vi "main.vi"() -> ()   [LabVIEW 2016]
uses:
  <vilib>/Utility/config.llb/Read Key (I32).vi
  <vilib>/Utility/config.llb/NI_LVConfig.lvlib
  <vilib>/httpClient/LabVIEWHTTPClient.lvlib
panel:
  out "QQ二维码路径":path
  out "webqq好友":string
  out "error out":errorcluster caption="错误输出"
  out "qqbat字符串":string
  out "心跳认证标志":bool
  in  "刷新时的PWM数值":dbl
  out "清扫模式记录数组":dbl[][](array[numeric])
  in  "刷新标志":bool
  out "测试布尔":bool
  out "起始秒":string
  out "起始小时":string
  out "文本已创建":bool
  out "修改定时数标志":bool
  out "错误输出 3":errorcluster caption="错误输出"
  out "布尔 2":bool
  out "清扫命令发出标志":bool
  in  "定时数":dbl=1.0
  out "图片路径":path
  in  "一直开灯":bool
  out "错误输出 2":errorcluster caption="错误输出"
  out "错误输出":errorcluster
  in  "开灯":bool
  in  "选项卡控件":T1(tab)
  in  "清扫模式选择开关":bool
  in  "清扫周期：":string="未运行"
  in  "清扫速度：":string="未运行"
  out "本机IP：":string
  out "控制器IP：":string
  in  "端口号：":i32=8848
  out "连接状态":bool
  in  "连接控制器":bool
  in  "确认定时":bool
  in  "清扫周期：":dbl(ring)=2.0 caption="清扫周期： 2" items=["2小时"=2.0, "4小时"=4.0, "6小时"=6.0, "8小时"=8.0, "10小时"=10.0, "12小时"=12.0, "14小时"=14.0]
  in  "清扫速度：":i32(slide) scale=1.0..10.0
  in  "清扫速度确认":bool
  in  "当前城市":string="杭州"
  out "天气：":string="未知"
  in  "等待：":i32=1000
  in  "断开连接":bool
  in  "确定当前城市":bool
  out "天气图标":T2
  out "滑动杆":T3 scale=0.0..100.0
  in  "清空接收区按钮":bool
  in  "待发送数据":string
  in  "发送按钮":bool
  out "数据接收显示":string="下列为接收到的数据..."
  in  "其他类清扫周期：":dbl(ring)=2.0 caption="清扫周期： 2" items=["2小时"=2.0, "4小时"=4.0, "6小时"=6.0, "8小时"=8.0, "10小时"=10.0, "12小时"=12.0, "14小时"=14.0]
  in  "其他类清扫速度：":i32(slide) scale=1.0..10.0
  in  "智能清扫模式确定按钮":bool
  in  "雨类清扫周期：":dbl(ring)=2.0 caption="清扫周期： 2" items=["2小时"=2.0, "4小时"=4.0, "6小时"=6.0, "8小时"=8.0, "10小时"=10.0, "12小时"=12.0, "14小时"=14.0]
  in  "雨类清扫速度：":i32(slide) scale=1.0..10.0
  in  "沙尘类清扫周期：":dbl(ring)=2.0 caption="清扫周期： 2" items=["2小时"=2.0, "4小时"=4.0, "6小时"=6.0, "8小时"=8.0, "10小时"=10.0, "12小时"=12.0, "14小时"=14.0]
  in  "沙尘类清扫速度：":i32(slide) scale=1.0..10.0
  in  "雪类清扫周期：":dbl(ring)=2.0 caption="清扫周期： 2" items=["2小时"=2.0, "4小时"=4.0, "6小时"=6.0, "8小时"=8.0, "10小时"=10.0, "12小时"=12.0, "14小时"=14.0]
  in  "雪类清扫速度：":i32(slide) scale=1.0..10.0
  in  "阴类清扫周期：":dbl(ring)=2.0 caption="清扫周期： 2" items=["2小时"=2.0, "4小时"=4.0, "6小时"=6.0, "8小时"=8.0, "10小时"=10.0, "12小时"=12.0, "14小时"=14.0]
  in  "阴类清扫速度：":i32(slide) scale=1.0..10.0
  in  "晴类清扫周期：":dbl(ring)=2.0 caption="清扫周期： 2" items=["2小时"=2.0, "4小时"=4.0, "6小时"=6.0, "8小时"=8.0, "10小时"=10.0, "12小时"=12.0, "14小时"=14.0]
  in  "晴类清扫速度：":i32(slide) scale=1.0..10.0
  in  "WebBrowser":refnum<k7>(container) caption="使用说明网页"
  in  "查看项目主页按钮":bool
  out "正在加载标志":T4
  in  "确认发送实时日志":bool
  out "QQ状态":bool
  out "接受者ID":string
  in  "搜索ID按钮":bool
  in  "接收者的QQ昵称或备注名":string
  in  "退出QQ号按钮":bool
  in  "打开QQ按钮":bool
  out "QQ登录二维码":picture
  out "发送返回值":string
  # "工作状态模拟"
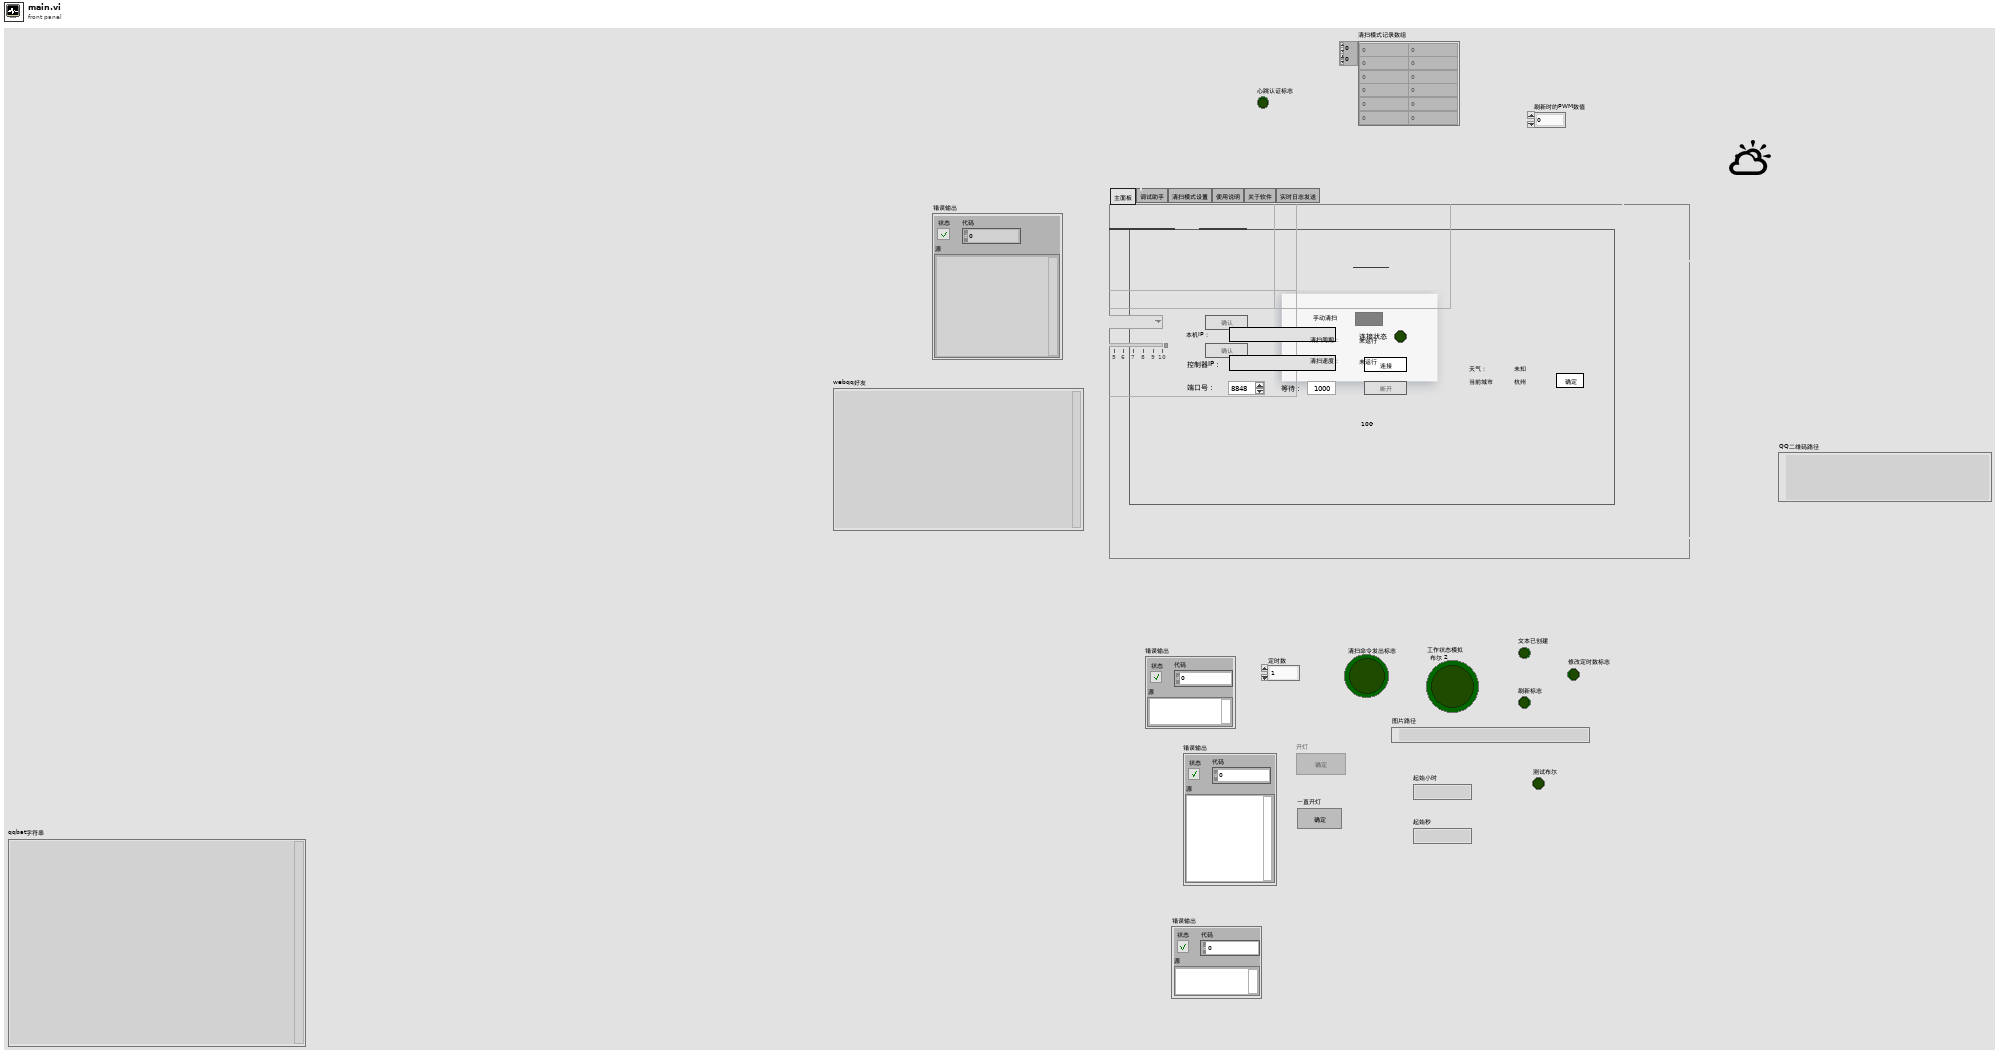
[diagram p1: front panel]
types:
  T1 = enum32{"主面板", "调试助手", "清扫模式设置", "使用说明", "关于软件", "实时日志发送"}
  T2 = typedef "透明背景.ctl" = picture
  T3 = typedef "背景控件.ctl" = dbl
  T4 = typedef "正在加载.ctl" = bool
  T5 = enum8{"Enabled", "Disabled", "Disabled and Grayed Out"}
  T6 = typedef "NI_LVConfig.lvlib/Config Data RefNum.ctl" = refnum<k1>
  T7 = typedef "LabVIEWHTTPClient.lvlib/ClientHandle.ctl" = refnum<k1>
  T8 = typedef "imagedata.ctl" = cluster{"image type":i32, "image depth":i32, "image":u8[], "mask":u8[], "colors":u32[], "Rectangle":cluster{"left":i16, "top":i16, "right":i16, "bottom":i16}}
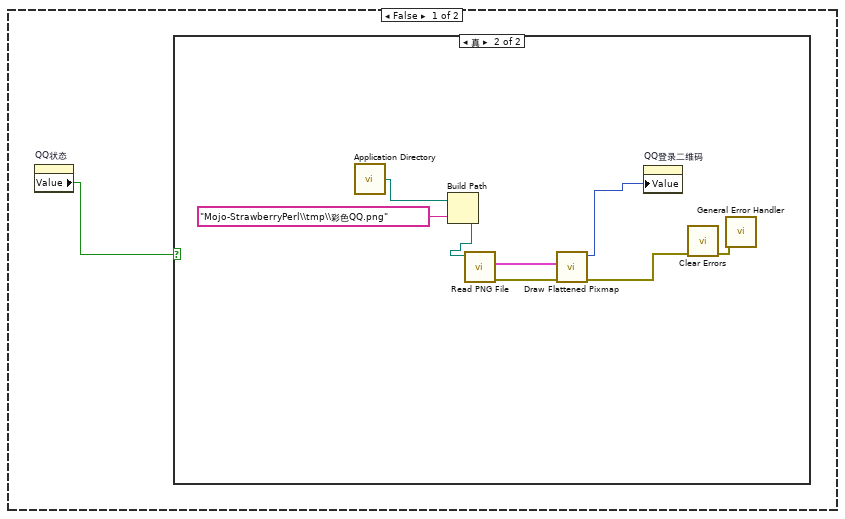
[diagram p2: hidden frame]
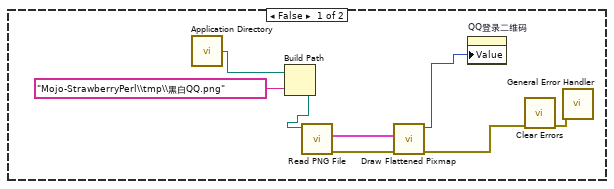
[diagram p3: hidden frame]
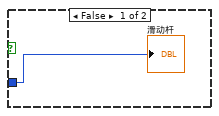
[diagram p5: hidden frame]
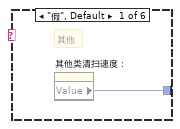
[diagram p8: hidden frame]
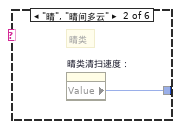
[diagram p9: hidden frame]
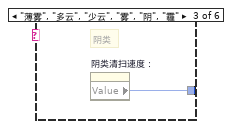
[diagram p10: hidden frame]
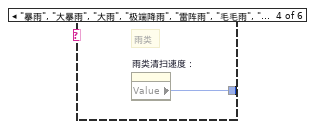
[diagram p11: hidden frame]
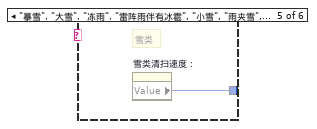
[diagram p12: hidden frame]
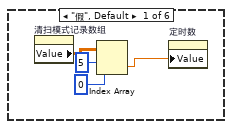
[diagram p14: hidden frame]
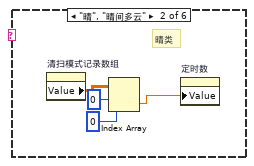
[diagram p15: hidden frame]
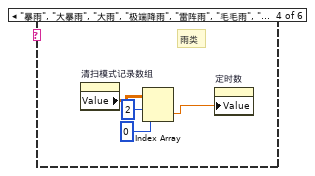
[diagram p16: hidden frame]
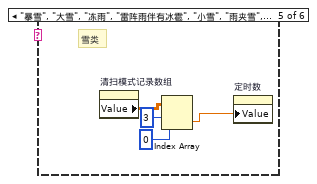
[diagram p17: hidden frame]
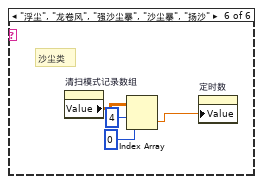
[diagram p18: hidden frame]
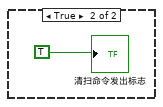
[diagram p20: hidden frame]
diagram:
  # "初始化"
  n1 = flat-sequence {
    frame #0 {
      w5 = T5."Disabled and Grayed Out" ("禁用")
      w34 = "" ("控制器IP：")
      n2 = property on="接收者的QQ昵称或备注名" class="Str"("Value"="" ("接收者的QQ昵称或备注名")) -> ()  [unwired: 2 in, 2 out]
      n3 = property on="接受者ID" class="Str"("Value"="" ("接受者ID")) -> ()  [unwired: 2 in, 2 out]
      n4 = property on="当前城市" class="Str"() -> ("Value"=w32:string)  [unwired: 2 in, 2 out]
      n5 = local write "连接状态"(FALSE ("连接状态")) -> ()
      n6 = Wait (ms)(milliseconds to wait=u32 10 ("等待时间（毫秒）")) -> ()  [unwired: 1 out]
      n7 = property on="QQ状态" class="Bool (严格)"("Value"=FALSE ("QQ状态")) -> ()  [unwired: 2 in, 2 out]
      n8 = property on="发送返回值" class="Str"("Value"="" ("发送返回值")) -> ()  [unwired: 2 in, 2 out]
      n9 = local write "本机IP："(w34) -> ()
      n10 = local write "控制器IP："(w34) -> ()
      n11 = property on="待发送数据" class="Str"("Value"="" ("待发送数据")) -> ()  [unwired: 2 in, 2 out]
      n12 = call "抓取天气查询.vi"("城市（市，县）"=w32) -> ("当前天气"=w31:string)
      n13 = property on="清扫速度：" class="Str"("Value"="未连接" ("清扫速度：")) -> ()  [unwired: 2 in, 2 out]
      n14 = property on="清扫周期：" class="Str"("Value"="未运行" ("清扫周期：")) -> ()  [unwired: 2 in, 2 out]
      n15 = call "获取时间.vi"() -> ("当前秒"=→"起始秒":string, "当前小时数"=→"起始小时":string)  [unwired: 8 in, 2 out]
      n16 = property on="天气：" class="Str"("Value"=w31) -> ()  [unwired: 2 in, 2 out]
      n17 = property on="连接控制器" class="Bool"("DisabledEnum"=T5."Enabled" ("禁用")) -> ()  [unwired: 2 in, 2 out]
      n18 = property on="正在加载标志" class="Bool (严格)"("Value"=FALSE ("获取好友标志")) -> ()  [unwired: 2 in, 2 out]
      n19 = property on="确认发送实时日志" class="Bool (严格)"("Value"=FALSE ("确认发送实时日志")) -> ()  [unwired: 2 in, 2 out]
      n20 = Concatenate Strings("和风天气图标\\" ("字符串"), "未知" ("字符串"), ".png" ("字符串")) -> (w25:string)
      n21 = property on="数据接收显示" class="Str"("Value"="下列为接收到的数据..." ("数据接收显示")) -> ()  [unwired: 2 in, 2 out]
      n22 = call <vilib>:"Application Directory.vi"() -> ("Application Directory"=w26:path)
      n23 = Initialize Array(0.0 ("元素"), 6 ("维数大小"), 2 ("维数大小")) -> (→"清扫模式记录数组":dbl[][])
      n24 = Build Path(base path=w26, name or relative path=w25) -> (appended path=w27:path)
      n25 = property on="开灯" class="Bool"("DisabledEnum"=w5) -> ()  [unwired: 2 in, 2 out]
      n26 = property on="智能清扫模式确定按钮" class="Bool"("DisabledEnum"=w5) -> ()  [unwired: 2 in, 2 out]
      n27 = property on="断开连接" class="Bool"("DisabledEnum"=w5) -> ()  [unwired: 2 in, 2 out]
      n28 = property on="发送按钮" class="Bool"("DisabledEnum"=w5) -> ()  [unwired: 2 in, 2 out]
      n29 = property on="清扫周期：" class="Ring (严格)"("DisabledEnum"=w5) -> ()  [unwired: 2 in, 2 out]
      n30 = property on="清扫速度：" class="Slide (严格)"("DisabledEnum"=w5) -> ()  [unwired: 2 in, 2 out]
      n31 = property on="确认定时" class="Bool"("DisabledEnum"=w5) -> ()  [unwired: 2 in, 2 out]
      n32 = property on="清扫速度确认" class="Bool"("DisabledEnum"=w5) -> ()  [unwired: 2 in, 2 out]
      n33 = property on="正在加载标志" class="Bool (严格)"("Visible"=FALSE ("可见")) -> ()  [unwired: 2 in, 2 out]
      n34 = property on="正在加载标志" class="Bool (严格)"("Value"=T4 FALSE ("正在加载标志")) -> ()  [unwired: 2 in, 2 out]
      n35 = property on="接收者的QQ昵称或备注名" class="Str"("DisabledEnum"=w5) -> ()  [unwired: 2 in, 2 out]
      n36 = property on="搜索ID按钮" class="Bool"("DisabledEnum"=w5) -> ()  [unwired: 2 in, 2 out]
      n37 = property on="确认发送实时日志" class="Bool (严格)"("DisabledEnum"=w5) -> ()  [unwired: 2 in, 2 out]
      n38 = property on="退出QQ号按钮" class="Bool"("DisabledEnum"=w5) -> ()  [unwired: 2 in, 2 out]
      n39 = call "显示图片.vi"("路径"=w27, "缩放因子"=1.1) -> ("二维图片"=w21:T2)  [unwired: 8 in]
      n40 = property on="天气图标" class="Pict (严格)"("Value"=w21) -> ()  [unwired: 2 in, 2 out]
    }
    frame #1 {
      n41 = call <vilib>:"Application Directory.vi"() -> ("Application Directory"=w46:path)
      n42 = Build Path(base path=w46, name or relative path="配置文件" ("名称或相对路径")) -> (appended path=w44:path)
      n43 = call <vilib>:"Open Config Data.vi"("create file if necessary (T)"=FALSE, "configuration file path"=w44) -> ("error out"=w36:errorcluster, "refnum"=w41:T6)  [unwired: 7 in, 1 out]
      n44 = call-poly <vilib>:"Read Key.vi"("section"="用户配置数据", "error in (no error)"=w36, "key"="端口号", "refnum"=w41) -> ("error out"=w37:errorcluster, "found?"=w38:bool)  [unwired: 4 in, 2 out]
      "文本已创建" <- w38
      n45 = case shown="真" w38 {
        frame False {
          n46 = call "保存配置.vi"() -> ()  [unwired: 20 in]
        }
        frame True {
        }
      }
      n47 = call <vilib>:"Clear Errors.vi"("error in (no error)"=w37) -> ("error out"=w42:errorcluster)  [unwired: 5 in, 1 out]
      n48 = call <vilib>:"General Error Handler.vi"("error in (no error)"=w42) -> ()  [unwired: 10 in, 5 out]
    }
    frame #2 {
      n49 = call "读取配置.vi"() -> ("端口号"=w51:i32, "等待"=w52:i32, "当前城市"=w53:string, "手动清扫周期"=w54:dbl, "手动清扫速度"=w55:i32, "清扫模式选择开关"=w56:bool, "晴类清扫周期"=w50:dbl, "阴类清扫周期"=w57:dbl, "雨类清扫周期"=w49:dbl, "雪类清扫周期"=w58:dbl, "沙尘类清扫周期"=w48:dbl, "其他类清扫周期"=w59:dbl, "晴类清扫速度"=w47:i32, "阴类清扫速度"=w60:i32, "雨类清扫速度"=w64:i32, "雪类清扫速度"=w63:i32, "沙尘类清扫速度"=w62:i32, "其他类清扫速度"=w61:i32)  [unwired: 2 in]
      n50 = property on="当前城市" class="Str"("Value"=w53) -> ()  [unwired: 2 in, 2 out]
      n51 = property on="等待：" class="DigNum (严格)"("Value"=w52) -> ()  [unwired: 2 in, 2 out]
      n52 = property on="端口号：" class="DigNum (严格)"("Value"=w51) -> ()  [unwired: 2 in, 2 out]
      n53 = property on="雪类清扫速度：" class="Slide (严格)"("Value"=w63) -> ()  [unwired: 2 in, 2 out]
      n54 = property on="沙尘类清扫速度：" class="Slide (严格)"("Value"=w62) -> ()  [unwired: 2 in, 2 out]
      n55 = property on="其他类清扫速度：" class="Slide (严格)"("Value"=w61) -> ()  [unwired: 2 in, 2 out]
      n56 = property on="阴类清扫速度：" class="Slide (严格)"("Value"=w60) -> ()  [unwired: 2 in, 2 out]
      n57 = property on="其他类清扫周期：" class="Ring (严格)"("Value"=w59) -> ()  [unwired: 2 in, 2 out]
      n58 = property on="雪类清扫周期：" class="Ring (严格)"("Value"=w58) -> ()  [unwired: 2 in, 2 out]
      n59 = property on="阴类清扫周期：" class="Ring (严格)"("Value"=w57) -> ()  [unwired: 2 in, 2 out]
      n60 = property on="清扫模式选择开关" class="Bool (严格)"("Value"=w56) -> ()  [unwired: 2 in, 2 out]
      n61 = property on="清扫速度：" class="Slide (严格)"("Value"=w55) -> ()  [unwired: 2 in, 2 out]
      n62 = property on="清扫周期：" class="Ring (严格)"("Value"=w54) -> ()  [unwired: 2 in, 2 out]
      n63 = property on="晴类清扫周期：" class="Ring (严格)"("Value"=w50) -> ()  [unwired: 2 in, 2 out]
      n64 = property on="雨类清扫周期：" class="Ring (严格)"("Value"=w49) -> ()  [unwired: 2 in, 2 out]
      n65 = property on="沙尘类清扫周期：" class="Ring (严格)"("Value"=w48) -> ()  [unwired: 2 in, 2 out]
      n66 = property on="晴类清扫速度：" class="Slide (严格)"("Value"=w47) -> ()  [unwired: 2 in, 2 out]
      n67 = property on="雨类清扫速度：" class="Slide (严格)"("Value"=w64) -> ()  [unwired: 2 in, 2 out]
    }
    frame #3 {
      w69 = 0 ("禁用的索引 (列)")
      w96 = 0 ("禁用的索引 (列)")
      w99 = 0 ("禁用的索引 (列)")
      w126 = 0 ("禁用的索引 (列)")
      w129 = 0 ("禁用的索引 (列)")
      w156 = 0 ("禁用的索引 (列)")
      w159 = 0 ("禁用的索引 (列)")
      w186 = 0 ("禁用的索引 (列)")
      w189 = 0 ("禁用的索引 (列)")
      w216 = 0 ("禁用的索引 (列)")
      w231 = 1 ("禁用的索引 (列)")
      # "获取本机IP地址"
      # "初始化天气图标"
      n68 = property on="天气：" class="Str"() -> ("Value"=w235:string)  [unwired: 2 in, 2 out]
      n69 = String To IP() -> (0:w66:u32)  [unwired: 1 in]
      n70 = String Length(string=w235) -> (length=w234:i32)
      n71 = IP To String(1:TRUE ("句点符号？(F)"), 2:w66) -> (0:→"本机IP：":string)
      n72 = property on="沙尘类清扫周期：" class="Ring (严格)"() -> ("Value"=w71:dbl)  [unwired: 2 in, 2 out]
      n73 = property on="沙尘类清扫周期：" class="Ring (严格)"() -> ("Value"=w94:dbl)  [unwired: 2 in, 2 out]
      n74 = property on="沙尘类清扫周期：" class="Ring (严格)"() -> ("Value"=w101:dbl)  [unwired: 2 in, 2 out]
      n75 = property on="沙尘类清扫周期：" class="Ring (严格)"() -> ("Value"=w124:dbl)  [unwired: 2 in, 2 out]
      n76 = property on="沙尘类清扫周期：" class="Ring (严格)"() -> ("Value"=w131:dbl)  [unwired: 2 in, 2 out]
      n77 = property on="沙尘类清扫周期：" class="Ring (严格)"() -> ("Value"=w154:dbl)  [unwired: 2 in, 2 out]
      n78 = property on="沙尘类清扫周期：" class="Ring (严格)"() -> ("Value"=w161:dbl)  [unwired: 2 in, 2 out]
      n79 = property on="沙尘类清扫周期：" class="Ring (严格)"() -> ("Value"=w184:dbl)  [unwired: 2 in, 2 out]
      n80 = property on="沙尘类清扫周期：" class="Ring (严格)"() -> ("Value"=w191:dbl)  [unwired: 2 in, 2 out]
      n81 = property on="沙尘类清扫周期：" class="Ring (严格)"() -> ("Value"=w214:dbl)  [unwired: 2 in, 2 out]
      n82 = Greater Than 0?(x=w234) -> (x > 0?=w233:bool)
      n83 = property on="雪类清扫周期：" class="Ring (严格)"() -> ("Value"=w73:dbl)  [unwired: 2 in, 2 out]
      n84 = property on="雪类清扫周期：" class="Ring (严格)"() -> ("Value"=w92:dbl)  [unwired: 2 in, 2 out]
      n85 = property on="雪类清扫周期：" class="Ring (严格)"() -> ("Value"=w103:dbl)  [unwired: 2 in, 2 out]
      n86 = property on="雪类清扫周期：" class="Ring (严格)"() -> ("Value"=w122:dbl)  [unwired: 2 in, 2 out]
      n87 = property on="雪类清扫周期：" class="Ring (严格)"() -> ("Value"=w133:dbl)  [unwired: 2 in, 2 out]
      n88 = property on="雪类清扫周期：" class="Ring (严格)"() -> ("Value"=w152:dbl)  [unwired: 2 in, 2 out]
      n89 = property on="雪类清扫周期：" class="Ring (严格)"() -> ("Value"=w163:dbl)  [unwired: 2 in, 2 out]
      n90 = property on="雪类清扫周期：" class="Ring (严格)"() -> ("Value"=w182:dbl)  [unwired: 2 in, 2 out]
      n91 = property on="雪类清扫周期：" class="Ring (严格)"() -> ("Value"=w193:dbl)  [unwired: 2 in, 2 out]
      n92 = property on="雪类清扫周期：" class="Ring (严格)"() -> ("Value"=w212:dbl)  [unwired: 2 in, 2 out]
      n93 = property on="雪类清扫速度：" class="Slide (严格)"() -> ("Value"=w227:i32)  [unwired: 2 in, 2 out]
      n94 = property on="晴类清扫速度：" class="Slide (严格)"() -> ("Value"=w221:i32)  [unwired: 2 in, 2 out]
      n95 = property on="阴类清扫速度：" class="Slide (严格)"() -> ("Value"=w223:i32)  [unwired: 2 in, 2 out]
      n96 = property on="雨类清扫速度：" class="Slide (严格)"() -> ("Value"=w225:i32)  [unwired: 2 in, 2 out]
      n97 = property on="沙尘类清扫速度：" class="Slide (严格)"() -> ("Value"=w229:i32)  [unwired: 2 in, 2 out]
      n98 = property on="雨类清扫周期：" class="Ring (严格)"() -> ("Value"=w75:dbl)  [unwired: 2 in, 2 out]
      n99 = property on="雨类清扫周期：" class="Ring (严格)"() -> ("Value"=w90:dbl)  [unwired: 2 in, 2 out]
      n100 = property on="雨类清扫周期：" class="Ring (严格)"() -> ("Value"=w105:dbl)  [unwired: 2 in, 2 out]
      n101 = property on="雨类清扫周期：" class="Ring (严格)"() -> ("Value"=w120:dbl)  [unwired: 2 in, 2 out]
      n102 = property on="雨类清扫周期：" class="Ring (严格)"() -> ("Value"=w135:dbl)  [unwired: 2 in, 2 out]
      n103 = property on="雨类清扫周期：" class="Ring (严格)"() -> ("Value"=w150:dbl)  [unwired: 2 in, 2 out]
      n104 = property on="雨类清扫周期：" class="Ring (严格)"() -> ("Value"=w165:dbl)  [unwired: 2 in, 2 out]
      n105 = property on="雨类清扫周期：" class="Ring (严格)"() -> ("Value"=w180:dbl)  [unwired: 2 in, 2 out]
      n106 = property on="雨类清扫周期：" class="Ring (严格)"() -> ("Value"=w195:dbl)  [unwired: 2 in, 2 out]
      n107 = property on="雨类清扫周期：" class="Ring (严格)"() -> ("Value"=w210:dbl)  [unwired: 2 in, 2 out]
      n108 = property on="其他类清扫周期：" class="Ring (严格)"() -> ("Value"=w68:dbl)  [unwired: 2 in, 2 out]
      n109 = property on="其他类清扫周期：" class="Ring (严格)"() -> ("Value"=w97:dbl)  [unwired: 2 in, 2 out]
      n110 = property on="其他类清扫周期：" class="Ring (严格)"() -> ("Value"=w98:dbl)  [unwired: 2 in, 2 out]
      n111 = property on="其他类清扫周期：" class="Ring (严格)"() -> ("Value"=w127:dbl)  [unwired: 2 in, 2 out]
      n112 = property on="其他类清扫周期：" class="Ring (严格)"() -> ("Value"=w128:dbl)  [unwired: 2 in, 2 out]
      n113 = property on="其他类清扫周期：" class="Ring (严格)"() -> ("Value"=w157:dbl)  [unwired: 2 in, 2 out]
      n114 = property on="其他类清扫周期：" class="Ring (严格)"() -> ("Value"=w158:dbl)  [unwired: 2 in, 2 out]
      n115 = property on="其他类清扫周期：" class="Ring (严格)"() -> ("Value"=w187:dbl)  [unwired: 2 in, 2 out]
      n116 = property on="其他类清扫周期：" class="Ring (严格)"() -> ("Value"=w188:dbl)  [unwired: 2 in, 2 out]
      n117 = property on="其他类清扫周期：" class="Ring (严格)"() -> ("Value"=w217:dbl)  [unwired: 2 in, 2 out]
      n118 = case shown="真" w233 {
        frame False {
        }
        frame True {
          n119 = property on="天气：" class="Str"() -> ("Value"=w236:string)  [unwired: 2 in, 2 out]
          n120 = Concatenate Strings("和风天气图标\\" ("字符串"), w236, ".png" ("字符串")) -> (w239:string)
          n121 = call <vilib>:"Application Directory.vi"() -> ("Application Directory"=w238:path)
          n122 = Build Path(base path=w238, name or relative path=w239) -> (appended path=w237:path)
          n123 = call "显示图片.vi"("路径"=w237, "缩放因子"=1.1) -> ("二维图片"=w243:T2)  [unwired: 8 in]
          n124 = property on="天气图标" class="Pict (严格)"("Value"=w243) -> ()  [unwired: 2 in, 2 out]
        }
      }
      n125 = property on="其他类清扫速度：" class="Slide (严格)"() -> ("Value"=w232:i32)  [unwired: 2 in, 2 out]
      n126 = property on="清扫模式记录数组" class="Arr (严格)"() -> ("Value"=w218:dbl[][])  [unwired: 2 in, 2 out]
      n127 = property on="阴类清扫周期：" class="Ring (严格)"() -> ("Value"=w77:dbl)  [unwired: 2 in, 2 out]
      n128 = property on="阴类清扫周期：" class="Ring (严格)"() -> ("Value"=w88:dbl)  [unwired: 2 in, 2 out]
      n129 = property on="阴类清扫周期：" class="Ring (严格)"() -> ("Value"=w107:dbl)  [unwired: 2 in, 2 out]
      n130 = property on="阴类清扫周期：" class="Ring (严格)"() -> ("Value"=w118:dbl)  [unwired: 2 in, 2 out]
      n131 = property on="阴类清扫周期：" class="Ring (严格)"() -> ("Value"=w137:dbl)  [unwired: 2 in, 2 out]
      n132 = property on="阴类清扫周期：" class="Ring (严格)"() -> ("Value"=w148:dbl)  [unwired: 2 in, 2 out]
      n133 = property on="阴类清扫周期：" class="Ring (严格)"() -> ("Value"=w167:dbl)  [unwired: 2 in, 2 out]
      n134 = property on="阴类清扫周期：" class="Ring (严格)"() -> ("Value"=w178:dbl)  [unwired: 2 in, 2 out]
      n135 = property on="阴类清扫周期：" class="Ring (严格)"() -> ("Value"=w197:dbl)  [unwired: 2 in, 2 out]
      n136 = property on="阴类清扫周期：" class="Ring (严格)"() -> ("Value"=w208:dbl)  [unwired: 2 in, 2 out]
      n137 = property on="晴类清扫周期：" class="Ring (严格)"() -> ("Value"=w81:dbl)  [unwired: 2 in, 2 out]
      n138 = property on="晴类清扫周期：" class="Ring (严格)"() -> ("Value"=w84:dbl)  [unwired: 2 in, 2 out]
      n139 = property on="晴类清扫周期：" class="Ring (严格)"() -> ("Value"=w111:dbl)  [unwired: 2 in, 2 out]
      n140 = property on="晴类清扫周期：" class="Ring (严格)"() -> ("Value"=w114:dbl)  [unwired: 2 in, 2 out]
      n141 = property on="晴类清扫周期：" class="Ring (严格)"() -> ("Value"=w141:dbl)  [unwired: 2 in, 2 out]
      n142 = property on="晴类清扫周期：" class="Ring (严格)"() -> ("Value"=w144:dbl)  [unwired: 2 in, 2 out]
      n143 = property on="晴类清扫周期：" class="Ring (严格)"() -> ("Value"=w171:dbl)  [unwired: 2 in, 2 out]
      n144 = property on="晴类清扫周期：" class="Ring (严格)"() -> ("Value"=w174:dbl)  [unwired: 2 in, 2 out]
      n145 = property on="晴类清扫周期：" class="Ring (严格)"() -> ("Value"=w201:dbl)  [unwired: 2 in, 2 out]
      n146 = property on="晴类清扫周期：" class="Ring (严格)"() -> ("Value"=w204:dbl)  [unwired: 2 in, 2 out]
      n147 = Replace Array Subset(array=w218, new element #1=w221, index (row) #1=0 ("索引 (行)"), index (col) #1=w231, new element #2=w223, index (row) #2=1 ("索引 (行)"), index (col) #2=w231, new element #3=w225, index (row) #3=2 ("索引 (行)"), index (col) #3=w231, new element #4=w227, index (row) #4=3 ("索引 (行)"), index (col) #4=w231, new element #5=w229, index (row) #5=4 ("索引 (行)"), index (col) #5=w231, new element #6=w232, index (row) #6=5 ("索引 (行)"), index (col) #6=w231) -> (w219:dbl[][])
      n148 = property on="清扫模式记录数组" class="Arr (严格)"() -> ("Value"=w82:dbl[][])  [unwired: 2 in, 2 out]
      n149 = property on="清扫模式记录数组" class="Arr (严格)"() -> ("Value"=w83:dbl[][])  [unwired: 2 in, 2 out]
      n150 = property on="清扫模式记录数组" class="Arr (严格)"() -> ("Value"=w112:dbl[][])  [unwired: 2 in, 2 out]
      n151 = property on="清扫模式记录数组" class="Arr (严格)"() -> ("Value"=w113:dbl[][])  [unwired: 2 in, 2 out]
      n152 = property on="清扫模式记录数组" class="Arr (严格)"() -> ("Value"=w142:dbl[][])  [unwired: 2 in, 2 out]
      n153 = property on="清扫模式记录数组" class="Arr (严格)"() -> ("Value"=w143:dbl[][])  [unwired: 2 in, 2 out]
      n154 = property on="清扫模式记录数组" class="Arr (严格)"() -> ("Value"=w172:dbl[][])  [unwired: 2 in, 2 out]
      n155 = property on="清扫模式记录数组" class="Arr (严格)"() -> ("Value"=w173:dbl[][])  [unwired: 2 in, 2 out]
      n156 = property on="清扫模式记录数组" class="Arr (严格)"() -> ("Value"=w202:dbl[][])  [unwired: 2 in, 2 out]
      n157 = property on="清扫模式记录数组" class="Arr (严格)"() -> ("Value"=w203:dbl[][])  [unwired: 2 in, 2 out]
      n158 = Replace Array Subset(array=w82, new element #1=w81, index (row) #1=0 ("索引 (行)"), index (col) #1=w69, new element #2=w77, index (row) #2=1 ("索引 (行)"), index (col) #2=w69, new element #3=w75, index (row) #3=2 ("索引 (行)"), index (col) #3=w69, new element #4=w73, index (row) #4=3 ("索引 (行)"), index (col) #4=w69, new element #5=w71, index (row) #5=4 ("索引 (行)"), index (col) #5=w69, new element #6=w68, index (row) #6=5 ("索引 (行)"), index (col) #6=w69) -> (w80:dbl[][])
      n159 = Replace Array Subset(array=w83, new element #1=w84, index (row) #1=0 ("索引 (行)"), index (col) #1=w96, new element #2=w88, index (row) #2=1 ("索引 (行)"), index (col) #2=w96, new element #3=w90, index (row) #3=2 ("索引 (行)"), index (col) #3=w96, new element #4=w92, index (row) #4=3 ("索引 (行)"), index (col) #4=w96, new element #5=w94, index (row) #5=4 ("索引 (行)"), index (col) #5=w96, new element #6=w97, index (row) #6=5 ("索引 (行)"), index (col) #6=w96) -> (w85:dbl[][])
      n160 = Replace Array Subset(array=w112, new element #1=w111, index (row) #1=0 ("索引 (行)"), index (col) #1=w99, new element #2=w107, index (row) #2=1 ("索引 (行)"), index (col) #2=w99, new element #3=w105, index (row) #3=2 ("索引 (行)"), index (col) #3=w99, new element #4=w103, index (row) #4=3 ("索引 (行)"), index (col) #4=w99, new element #5=w101, index (row) #5=4 ("索引 (行)"), index (col) #5=w99, new element #6=w98, index (row) #6=5 ("索引 (行)"), index (col) #6=w99) -> (w110:dbl[][])
      n161 = Replace Array Subset(array=w113, new element #1=w114, index (row) #1=0 ("索引 (行)"), index (col) #1=w126, new element #2=w118, index (row) #2=1 ("索引 (行)"), index (col) #2=w126, new element #3=w120, index (row) #3=2 ("索引 (行)"), index (col) #3=w126, new element #4=w122, index (row) #4=3 ("索引 (行)"), index (col) #4=w126, new element #5=w124, index (row) #5=4 ("索引 (行)"), index (col) #5=w126, new element #6=w127, index (row) #6=5 ("索引 (行)"), index (col) #6=w126) -> (w115:dbl[][])
      n162 = Replace Array Subset(array=w142, new element #1=w141, index (row) #1=0 ("索引 (行)"), index (col) #1=w129, new element #2=w137, index (row) #2=1 ("索引 (行)"), index (col) #2=w129, new element #3=w135, index (row) #3=2 ("索引 (行)"), index (col) #3=w129, new element #4=w133, index (row) #4=3 ("索引 (行)"), index (col) #4=w129, new element #5=w131, index (row) #5=4 ("索引 (行)"), index (col) #5=w129, new element #6=w128, index (row) #6=5 ("索引 (行)"), index (col) #6=w129) -> (w140:dbl[][])
      n163 = Replace Array Subset(array=w143, new element #1=w144, index (row) #1=0 ("索引 (行)"), index (col) #1=w156, new element #2=w148, index (row) #2=1 ("索引 (行)"), index (col) #2=w156, new element #3=w150, index (row) #3=2 ("索引 (行)"), index (col) #3=w156, new element #4=w152, index (row) #4=3 ("索引 (行)"), index (col) #4=w156, new element #5=w154, index (row) #5=4 ("索引 (行)"), index (col) #5=w156, new element #6=w157, index (row) #6=5 ("索引 (行)"), index (col) #6=w156) -> (w145:dbl[][])
      n164 = Replace Array Subset(array=w172, new element #1=w171, index (row) #1=0 ("索引 (行)"), index (col) #1=w159, new element #2=w167, index (row) #2=1 ("索引 (行)"), index (col) #2=w159, new element #3=w165, index (row) #3=2 ("索引 (行)"), index (col) #3=w159, new element #4=w163, index (row) #4=3 ("索引 (行)"), index (col) #4=w159, new element #5=w161, index (row) #5=4 ("索引 (行)"), index (col) #5=w159, new element #6=w158, index (row) #6=5 ("索引 (行)"), index (col) #6=w159) -> (w170:dbl[][])
      n165 = Replace Array Subset(array=w173, new element #1=w174, index (row) #1=0 ("索引 (行)"), index (col) #1=w186, new element #2=w178, index (row) #2=1 ("索引 (行)"), index (col) #2=w186, new element #3=w180, index (row) #3=2 ("索引 (行)"), index (col) #3=w186, new element #4=w182, index (row) #4=3 ("索引 (行)"), index (col) #4=w186, new element #5=w184, index (row) #5=4 ("索引 (行)"), index (col) #5=w186, new element #6=w187, index (row) #6=5 ("索引 (行)"), index (col) #6=w186) -> (w175:dbl[][])
      n166 = Replace Array Subset(array=w202, new element #1=w201, index (row) #1=0 ("索引 (行)"), index (col) #1=w189, new element #2=w197, index (row) #2=1 ("索引 (行)"), index (col) #2=w189, new element #3=w195, index (row) #3=2 ("索引 (行)"), index (col) #3=w189, new element #4=w193, index (row) #4=3 ("索引 (行)"), index (col) #4=w189, new element #5=w191, index (row) #5=4 ("索引 (行)"), index (col) #5=w189, new element #6=w188, index (row) #6=5 ("索引 (行)"), index (col) #6=w189) -> (w200:dbl[][])
      n167 = Replace Array Subset(array=w203, new element #1=w204, index (row) #1=0 ("索引 (行)"), index (col) #1=w216, new element #2=w208, index (row) #2=1 ("索引 (行)"), index (col) #2=w216, new element #3=w210, index (row) #3=2 ("索引 (行)"), index (col) #3=w216, new element #4=w212, index (row) #4=3 ("索引 (行)"), index (col) #4=w216, new element #5=w214, index (row) #5=4 ("索引 (行)"), index (col) #5=w216, new element #6=w217, index (row) #6=5 ("索引 (行)"), index (col) #6=w216) -> (w205:dbl[][])
      n168 = property on="清扫模式记录数组" class="Arr (严格)"("Value"=w219) -> ()  [unwired: 2 in, 2 out]
      n169 = property on="清扫模式记录数组" class="Arr (严格)"("Value"=w80) -> ()  [unwired: 2 in, 2 out]
      n170 = property on="清扫模式记录数组" class="Arr (严格)"("Value"=w85) -> ()  [unwired: 2 in, 2 out]
      n171 = property on="清扫模式记录数组" class="Arr (严格)"("Value"=w110) -> ()  [unwired: 2 in, 2 out]
      n172 = property on="清扫模式记录数组" class="Arr (严格)"("Value"=w115) -> ()  [unwired: 2 in, 2 out]
      n173 = property on="清扫模式记录数组" class="Arr (严格)"("Value"=w140) -> ()  [unwired: 2 in, 2 out]
      n174 = property on="清扫模式记录数组" class="Arr (严格)"("Value"=w145) -> ()  [unwired: 2 in, 2 out]
      n175 = property on="清扫模式记录数组" class="Arr (严格)"("Value"=w170) -> ()  [unwired: 2 in, 2 out]
      n176 = property on="清扫模式记录数组" class="Arr (严格)"("Value"=w175) -> ()  [unwired: 2 in, 2 out]
      n177 = property on="清扫模式记录数组" class="Arr (严格)"("Value"=w200) -> ()  [unwired: 2 in, 2 out]
      n178 = property on="清扫模式记录数组" class="Arr (严格)"("Value"=w205) -> ()  [unwired: 2 in, 2 out]
    }
  }
  n179 = while {
    shift-right: [w244] -> w1
    shift-left: refnum<k5> refnum ("connection ID") -> [w266]
    stop <- FALSE stop-if-true
    # "读取TCP数据"
    n180 = event shown="[2] \"打开QQ按钮\": 值改变" {
      selector: _ -> [_ _ _ _ _ _ _ _ _ _ _ _ _ _ _ _]
      dyn-events: _ -> [_ _ _ _ _ _ _ _ _ _ _ _ _ _ _ _]
      timeout: 50 -> [_ _ _ _ _ _ _ _ _ _ _ _ _ _ _ _]
      tunnel: w266 -> [w376 w379 _ _ _ _ w543 w551 w616 w621 w627 w629 w630 w639 w700 w715]
      tunnel: [w376 w377 _ _ _ _ w544 w550 w615 w618 w627 w629 w630 w638 w698 w714] -> w259
      tunnel: [_ _ _ _ _ _ _ _ w614 _ _ _ _ _ w699 w713] -> w258
      event Timeout {
        n181 = event-data() -> ()  [unwired: 1 in, 3 out]
      }
      event "连接控制器": Value Change {
        n182 = event-data() -> ()  [unwired: 1 in, 6 out]
        n183 = flat-sequence {
          tunnel: [w405] -> w380
          tunnel: [w404] -> w378
          tunnel: w379 -> [w395]
          frame #0 {
            w382 = T5."Disabled and Grayed Out" ("禁用")
            n184 = stacked-sequence {
              frame #0 {
                n185 = property on="当前城市" class="Str"() -> ("Value"=w386:string)  [unwired: 2 in, 2 out]
                n186 = call "抓取天气查询.vi"("城市（市，县）"=w386) -> ("当前天气"=w385:string)
                n187 = property on="天气：" class="Str"("Value"=w385) -> ()  [unwired: 2 in, 2 out]
              }
              frame #1 {
                n188 = call <vilib>:"Application Directory.vi"() -> ("Application Directory"=w394:path)
                n189 = property on="天气：" class="Str"() -> ("Value"=w387:string)  [unwired: 2 in, 2 out]
                n190 = Concatenate Strings("和风天气图标\\" ("字符串"), w387, ".png" ("字符串")) -> (w392:string)
                n191 = Build Path(base path=w394, name or relative path=w392) -> (appended path=w393:path)
                n192 = call "显示图片.vi"("路径"=w393, "缩放因子"=1.1) -> ("二维图片"=w388:T2)  [unwired: 8 in]
                n193 = property on="天气图标" class="Pict (严格)"("Value"=w388) -> ()  [unwired: 2 in, 2 out]
              }
            }
            n194 = property on="连接状态" class="Bool (严格)"("Value"=FALSE ("连接状态")) -> ()  [unwired: 2 in, 2 out]
            n195 = property on="清扫周期：" class="Str"("Value"="未运行" ("清扫周期：")) -> ()  [unwired: 2 in, 2 out]
            n196 = local write "控制器IP："("" ("控制器IP：")) -> ()
            n197 = property on="发送按钮" class="Bool"("DisabledEnum"=w382) -> ()  [unwired: 2 in, 2 out]
            n198 = property on="清扫速度确认" class="Bool"("DisabledEnum"=w382) -> ()  [unwired: 2 in, 2 out]
            n199 = property on="确认定时" class="Bool"("DisabledEnum"=w382) -> ()  [unwired: 2 in, 2 out]
            n200 = property on="开灯" class="Bool"("DisabledEnum"=w382) -> ()  [unwired: 2 in, 2 out]
            n201 = property on="连接控制器" class="Bool"("DisabledEnum"=w382) -> ()  [unwired: 2 in, 2 out]
          }
          frame #1 {
            n202 = call <vilib>:"TCP Listen.vi"("timeout ms (wait forever: -1)"="等待：", "port"="端口号：") -> ("error out"=w399:errorcluster, "remote address"=→"控制器IP：":string, "connection ID"=w404:refnum<k5>)  [unwired: 5 in, 2 out]
            n203 = Unbundle By Name(w399) -> ("status"=w396:bool)
            "布尔 2" <- w396
            n204 = case shown="真" w396 {
              tunnel: w395 -> [_ w408]
              frame False {
              }
              frame True {
                n205 = One Button Dialog(message="在等待时间内未连接上\n请确认端口号是否正确\n或机器是否已正确连接" ("消息"), button name ("OK")="好的我检查一下" ("T按钮名称（“确定”）")) -> (true=w409:bool)
                n206 = case shown="真" w409 {
                  tunnel: w408 -> [_ w410]
                  frame False {
                  }
                  frame True {
                    n207 = flat-sequence {
                      tunnel: w410 -> [w412]
                      frame #0 {
                        n208 = TCP Close Connection(connection ID=w412) -> (error out=→"错误输出 3":errorcluster)  [unwired: 2 in, 1 out]
                      }
                      frame #1 {
                        w413 = T5."Disabled and Grayed Out" ("禁用")
                        n209 = local write "控制器IP："("" ("控制器IP：")) -> ()
                        n210 = local write "连接状态"(FALSE ("连接状态")) -> ()
                        n211 = property on="连接控制器" class="Bool"("DisabledEnum"=T5."Enabled" ("禁用")) -> ()  [unwired: 2 in, 2 out]
                        n212 = property on="确认定时" class="Bool"("DisabledEnum"=w413) -> ()  [unwired: 2 in, 2 out]
                        n213 = property on="清扫速度确认" class="Bool"("DisabledEnum"=w413) -> ()  [unwired: 2 in, 2 out]
                        n214 = property on="开灯" class="Bool"("DisabledEnum"=w413) -> ()  [unwired: 2 in, 2 out]
                        n215 = property on="发送按钮" class="Bool"("DisabledEnum"=w413) -> ()  [unwired: 2 in, 2 out]
                        n216 = property on="断开连接" class="Bool"("DisabledEnum"=w413) -> ()  [unwired: 2 in, 2 out]
                      }
                    }
                  }
                }
              }
            }
            n217 = Not(x=w396) -> (.not. x?=w400:bool)
            n218 = Not A Number/Path/Refnum?(number/path/refnum=w404) -> (NaN/Path/Refnum?=w398:bool)
            n219 = Not(x=w398) -> (.not. x?=w397:bool)
            n220 = And(x=w397, y=w400) -> (x .and. y?=w405:bool)
          }
        }
        n221 = case shown="真" w380 {
          tunnel: w378 -> [w417 w419]
          tunnel: [w417 w418] -> w377
          frame False {
          }
          frame True {
            w421 = T5."Enabled" ("禁用")
            # "智能清扫为ON/真"
            # "恢复按钮使用权限"
            n222 = property on="清扫模式选择开关" class="Bool (严格)"() -> ("Value"=w420:bool)  [unwired: 2 in, 2 out]
            n223 = case shown="真" w420 {
              tunnel: [w429 w448] -> w418
              tunnel: w419 -> [w428 w449]
              frame False {
                w424 = T5."Enabled" ("禁用")
                # "手动清扫模式"
                n224 = property on="清扫速度：" class="Slide (严格)"() -> ("Value"=w433:i32)  [unwired: 2 in, 2 out]
                n225 = formula code="Y=X*15+105;"("X"=w433) -> ("Y"=w432:dbl)
                n226 = property on="智能清扫模式确定按钮" class="Bool"("DisabledEnum"=T5."Disabled and Grayed Out" ("禁用")) -> ()  [unwired: 2 in, 2 out]
                n227 = property on="清扫速度确认" class="Bool"("DisabledEnum"=w424) -> ()  [unwired: 2 in, 2 out]
                n228 = Number To Decimal String(number=w432) -> (decimal integer string=w430:string)  [unwired: 1 in]
                n229 = property on="确认定时" class="Bool"("DisabledEnum"=w424) -> ()  [unwired: 2 in, 2 out]
                n230 = property on="清扫周期：" class="Ring (严格)"("DisabledEnum"=w424) -> ()  [unwired: 2 in, 2 out]
                n231 = property on="清扫速度：" class="Slide (严格)"("DisabledEnum"=w424) -> ()  [unwired: 2 in, 2 out]
                n232 = Concatenate Strings("pwm" ("字符串"), w430) -> (w425:string)
                n233 = flat-sequence {
                  frame #0 {
                    n234 = property on="清扫周期：" class="Ring (严格)"() -> ("Value"=w434:dbl)  [unwired: 2 in, 2 out]
                    n235 = property on="定时数" class="DigNum (严格)"("Value"=w434) -> ()  [unwired: 2 in, 2 out]
                  }
                  frame #1 {
                    n236 = property on="定时数" class="DigNum (严格)"() -> ("Value"=w439:dbl)  [unwired: 2 in, 2 out]
                    n237 = Number To Fractional String(number=w439, precision (6)=i16 1 ("精度(6)")) -> (F-format string=w437:string)  [unwired: 2 in]
                    n238 = Concatenate Strings(w437, "小时" ("字符串")) -> (w436:string)
                    n239 = property on="清扫周期：" class="Str"("Value"=w436) -> ()  [unwired: 2 in, 2 out]
                  }
                }
                n240 = property on="清扫速度：" class="Str"("Value"=w425) -> ()  [unwired: 2 in, 2 out]
                n241 = TCP Write(connection ID=w428, data in=w425) -> (connection ID out=w429:refnum<k5>, error out=w427:errorcluster)  [unwired: 2 in, 1 out]
                n242 = call <vilib>:"Clear Errors.vi"("error in (no error)"=w427) -> ("error out"=w426:errorcluster)  [unwired: 5 in, 1 out]
                n243 = call <vilib>:"Simple Error Handler.vi"("error in (no error)"=w426) -> ()  [unwired: 4 in, 5 out]
              }
              frame True {
                w451 = T5."Disabled and Grayed Out" ("禁用")
                # "智能清扫模式"
                n244 = property on="天气：" class="Str"() -> ("Value"=w447:string)  [unwired: 2 in, 2 out]
                n245 = case shown="\"浮尘\", \"龙卷风\", \"强沙尘暴\", \"沙尘暴\", \"扬沙\"" w447 {
                  tunnel: [w452 w453 w454 w455 w456 w457] -> w440
                  frame "假", Default {
                    # "其他"
                    n246 = property on="其他类清扫速度：" class="Slide (严格)"() -> ("Value"=w452:i32)  [unwired: 2 in, 2 out]
                  }
                  frame "晴", "晴间多云" {
                    # "晴类"
                    n247 = property on="晴类清扫速度：" class="Slide (严格)"() -> ("Value"=w453:i32)  [unwired: 2 in, 2 out]
                  }
                  frame "薄雾", "多云", "少云", "雾", "阴", "霾" {
                    # "阴类"
                    n248 = property on="阴类清扫速度：" class="Slide (严格)"() -> ("Value"=w454:i32)  [unwired: 2 in, 2 out]
                  }
                  frame "暴雨", "大暴雨", "大雨", "极端降雨", "雷阵雨", "毛毛雨", "强雷阵雨", "强阵雨", "特大暴雨", "细雨", "小雨", "阵雨", "中雨" {
                    # "雨类"
                    n249 = property on="雨类清扫速度：" class="Slide (严格)"() -> ("Value"=w455:i32)  [unwired: 2 in, 2 out]
                  }
                  frame "暴雪", "大雪", "冻雨", "雷阵雨伴有冰雹", "小雪", "雨夹雪", "雨雪天气", "阵雪", "阵雨夹雪", "中雪" {
                    # "雪类"
                    n250 = property on="雪类清扫速度：" class="Slide (严格)"() -> ("Value"=w456:i32)  [unwired: 2 in, 2 out]
                  }
                  frame "浮尘", "龙卷风", "强沙尘暴", "沙尘暴", "扬沙" {
                    # "沙尘类"
                    n251 = property on="沙尘类清扫速度：" class="Slide (严格)"() -> ("Value"=w457:i32)  [unwired: 2 in, 2 out]
                  }
                }
                n252 = property on="智能清扫模式确定按钮" class="Bool"("DisabledEnum"=T5."Enabled" ("禁用")) -> ()  [unwired: 2 in, 2 out]
                n253 = property on="确认定时" class="Bool"("DisabledEnum"=w451) -> ()  [unwired: 2 in, 2 out]
                n254 = property on="清扫速度确认" class="Bool"("DisabledEnum"=w451) -> ()  [unwired: 2 in, 2 out]
                n255 = flat-sequence {
                  frame #0 {
                    # "处理清扫周期"
                    n256 = property on="天气：" class="Str"() -> ("Value"=w458:string)  [unwired: 2 in, 2 out]
                    n257 = case shown="\"薄雾\", \"多云\", \"少云\", \"雾\", \"阴\", \"霾\"" w458 {
                      frame "假", Default {
                        n258 = property on="其他类清扫周期：" class="Ring (严格)"() -> ("Value"=w459:dbl)  [unwired: 2 in, 2 out]
                        n259 = property on="定时数" class="DigNum (严格)"("Value"=w459) -> ()  [unwired: 2 in, 2 out]
                      }
                      frame "晴", "晴间多云" {
                        # "晴类"
                        n260 = property on="晴类清扫周期：" class="Ring (严格)"() -> ("Value"=w460:dbl)  [unwired: 2 in, 2 out]
                        n261 = property on="定时数" class="DigNum (严格)"("Value"=w460) -> ()  [unwired: 2 in, 2 out]
                      }
                      frame "薄雾", "多云", "少云", "雾", "阴", "霾" {
                        # "阴类"
                        n262 = property on="阴类清扫周期：" class="Ring (严格)"() -> ("Value"=w461:dbl)  [unwired: 2 in, 2 out]
                        n263 = property on="定时数" class="DigNum (严格)"("Value"=w461) -> ()  [unwired: 2 in, 2 out]
                      }
                      frame "暴雨", "大暴雨", "大雨", "极端降雨", "雷阵雨", "毛毛雨", "强雷阵雨", "强阵雨", "特大暴雨", "细雨", "小雨", "阵雨", "中雨" {
                        # "雨类"
                        n264 = property on="雨类清扫周期：" class="Ring (严格)"() -> ("Value"=w462:dbl)  [unwired: 2 in, 2 out]
                        n265 = property on="定时数" class="DigNum (严格)"("Value"=w462) -> ()  [unwired: 2 in, 2 out]
                      }
                      frame "暴雪", "大雪", "冻雨", "雷阵雨伴有冰雹", "小雪", "雨夹雪", "雨雪天气", "阵雪", "阵雨夹雪", "中雪" {
                        # "雪类"
                        n266 = property on="雪类清扫周期：" class="Ring (严格)"() -> ("Value"=w463:dbl)  [unwired: 2 in, 2 out]
                        n267 = property on="定时数" class="DigNum (严格)"("Value"=w463) -> ()  [unwired: 2 in, 2 out]
                      }
                      frame "浮尘", "龙卷风", "强沙尘暴", "沙尘暴", "扬沙" {
                        # "沙尘类"
                        n268 = property on="沙尘类清扫周期：" class="Ring (严格)"() -> ("Value"=w464:dbl)  [unwired: 2 in, 2 out]
                        n269 = property on="定时数" class="DigNum (严格)"("Value"=w464) -> ()  [unwired: 2 in, 2 out]
                      }
                    }
                  }
                  frame #1 {
                    n270 = property on="定时数" class="DigNum (严格)"() -> ("Value"=w469:dbl)  [unwired: 2 in, 2 out]
                    n271 = Number To Fractional String(number=w469, precision (6)=i16 1 ("精度(6)")) -> (F-format string=w467:string)  [unwired: 2 in]
                    n272 = Concatenate Strings(w467, "小时" ("字符串")) -> (w466:string)
                    n273 = property on="清扫周期：" class="Str"("Value"=w466) -> ()  [unwired: 2 in, 2 out]
                  }
                }
                n274 = formula code="Y=X*15+105;"("X"=w440) -> ("Y"=w446:dbl)
                n275 = Number To Decimal String(number=w446) -> (decimal integer string=w444:string)  [unwired: 1 in]
                n276 = Concatenate Strings("pwm" ("字符串"), w444) -> (w441:string)
                n277 = property on="清扫速度：" class="Str"("Value"=w441) -> ()  [unwired: 2 in, 2 out]
                n278 = TCP Write(connection ID=w449, data in=w441) -> (connection ID out=w448:refnum<k5>, error out=w443:errorcluster)  [unwired: 2 in, 1 out]
                n279 = call <vilib>:"Clear Errors.vi"("error in (no error)"=w443) -> ("error out"=w442:errorcluster)  [unwired: 5 in, 1 out]
                n280 = call <vilib>:"Simple Error Handler.vi"("error in (no error)"=w442) -> ()  [unwired: 4 in, 5 out]
              }
            }
            n281 = property on="断开连接" class="Bool"("DisabledEnum"=w421) -> ()  [unwired: 2 in, 2 out]
            n282 = property on="开灯" class="Bool"("DisabledEnum"=w421) -> ()  [unwired: 2 in, 2 out]
            n283 = property on="发送按钮" class="Bool"("DisabledEnum"=w421) -> ()  [unwired: 2 in, 2 out]
            "连接状态" <- TRUE ("控制器状态指示")
          }
        }
      }
      event "打开QQ按钮": Value Change {
        n284 = event-data() -> ()  [unwired: 1 in, 6 out]
        n285 = stacked-sequence {
          frame #0 {
            n286 = call <vilib>:"Application Directory.vi"() -> ("Application Directory"=w471:path)
            n287 = Build Path(base path=w471, name or relative path="Mojo-StrawberryPerl\\" ("名称或相对路径")) -> (appended path=w470:path)
            n288 = Build Path(base path=w470, name or relative path="start_mojo_webqq.bat" ("名称或相对路径")) -> (appended path=w476:path)
            n289 = Path To String(path=w476) -> (string=w477:string)
            n290 = call <vilib>:"System Exec.vi"("wait until completion? (T)"=FALSE, "working directory"=w470, "command line"=w477) -> ("error out"=→"error out":errorcluster, "standard output"=→"qqbat字符串":string)  [unwired: 5 in, 2 out]
          }
          frame #1 {
            n291 = property on="正在加载标志" class="Bool (严格)"("Value"=TRUE ("获取好友标志")) -> ()  [unwired: 2 in, 2 out]
            n292 = property on="正在加载标志" class="Bool (严格)"("Visible"=TRUE ("可见")) -> ()  [unwired: 2 in, 2 out]
          }
        }
      }
      event "搜索ID按钮": Value Change {
        n293 = event-data() -> ()  [unwired: 1 in, 6 out]
        n294 = flat-sequence {
          frame #0 {
            n295 = Concatenate Strings("http://127.0.0.1:5000/openqq/get_friend_info" ("字符串")) -> (w486:string)
            n296 = call <vilib>:"OpenHandle.vi"() -> ("client handle out"=w491:T7)  [unwired: 14 in, 1 out]
            n297 = Text to UTF-8(11:w486) -> (3:w488:string)  [unwired: 2 in, 1 out]
            n298 = call <vilib>:"GET.vi"("client handle"=w491, "url"=w488) -> ("client handle out"=w490:T7, "body"=w489:string, "error out"=w485:errorcluster)  [unwired: 10 in, 1 out]
            n299 = call <vilib>:"Clear Errors.vi"("error in (no error)"=w485) -> ("error out"=w484:errorcluster)  [unwired: 5 in, 1 out]
            n300 = call <vilib>:"CloseHandle.vi"("client handle"=w490) -> ()  [unwired: 14 in, 1 out]
            n301 = call <vilib>:"General Error Handler.vi"("error in (no error)"=w484) -> ()  [unwired: 10 in, 5 out]
            n302 = UTF-8 to Text(11:w489) -> (3:w482:string)  [unwired: 2 in, 1 out]
            "webqq好友" <- w482
            n303 = String Length(string=w482) -> (length=w483:i32)
            n304 = Greater Than 0?(x=w483) -> (x > 0?=w481:bool)
            n305 = case shown="真" w481 {
              frame False {
              }
              frame True {
                n306 = property on="接收者的QQ昵称或备注名" class="Str"() -> ("Value"=w494:string)  [unwired: 2 in, 2 out]
                n307 = property on="webqq好友" class="Str"() -> ("Value"=w495:string)  [unwired: 2 in, 2 out]
                n308 = Search and Replace String(replace all?=TRUE ("替换全部？(F)"), input string=w495, search string=w494) -> (number of replacements=w493:i32)  [unwired: 5 in, 3 out]
                n309 = Greater Than 0?(x=w493) -> (x > 0?=w492:bool)
                n310 = case shown="真" w492 {
                  frame False {
                  }
                  frame True {
                    n311 = property on="webqq好友" class="Str"() -> ("Value"=w500:string)  [unwired: 2 in, 2 out]
                    n312 = property on="接收者的QQ昵称或备注名" class="Str"() -> ("Value"=w499:string)  [unwired: 2 in, 2 out]
                    n313 = Match Pattern(string=w500, regular expression=w499) -> (before substring=w497:string)  [unwired: 1 in, 3 out]
                    n314 = Search and Replace String(replace all?=TRUE ("替换全部？(F)"), input string=w497, search string="\"id\"" ("搜索字符串")) -> (number of replacements=w498:i32)  [unwired: 5 in, 3 out]
                    n315 = for {
                      N: w498 -> [w506]
                      shift-right: [w503] -> _
                      shift-left: w497 -> [w504]
                      i -> [w508]
                      n316 = Decrement(x=w506) -> (x-1=w505:i32)
                      n317 = Equal?(x=w508, y=w505) -> (x = y?=w507:bool)
                      n318 = Match Pattern(string=w504, regular expression="\"id\":" ("正则表达式")) -> (after substring=w503:string)  [unwired: 1 in, 3 out]
                      n319 = case shown="真" w507 {
                        tunnel: w503 -> [_ w511]
                        frame False {
                        }
                        frame True {
                          n320 = Match Pattern(string=w511, regular expression="," ("正则表达式")) -> (before substring=→"接受者ID":string)  [unwired: 1 in, 3 out]
                        }
                      }
                    }
                  }
                }
              }
            }
          }
          frame #1 {
          }
        }
      }
      event "退出QQ号按钮": Value Change {
        n321 = event-data() -> ()  [unwired: 1 in, 6 out]
        n322 = stacked-sequence {
          frame #0 {
            n323 = property on="正在加载标志" class="Bool (严格)"("Value"=FALSE ("获取好友标志")) -> ()  [unwired: 2 in, 2 out]
            n324 = property on="QQ状态" class="Bool (严格)"("Value"=FALSE ("QQ状态")) -> ()  [unwired: 2 in, 2 out]
            n325 = property on="webqq好友" class="Str"() -> ("Value"=w523:string)  [unwired: 2 in, 2 out]
            n326 = Match Pattern(string=w523, regular expression="\"id\":" ("正则表达式")) -> (after substring=w531:string)  [unwired: 1 in, 3 out]
            n327 = call <vilib>:"Application Directory.vi"() -> ("Application Directory"=w513:path)
            n328 = call <vilib>:"Application Directory.vi"() -> ("Application Directory"=w520:path)
            n329 = Match Pattern(string=w531, regular expression="," ("正则表达式")) -> (before substring=w533:string)  [unwired: 1 in, 3 out]
            n330 = Build Path(base path=w513, name or relative path="Mojo-StrawberryPerl\\tmp\\mojo_webqq_cookie_default.dat" ("名称或相对路径")) -> (appended path=w515:path)
            n331 = Build Path(base path=w520, name or relative path="Mojo-StrawberryPerl\\tmp\\mojo_webqq_state_default.json" ("名称或相对路径")) -> (appended path=w518:path)
            n332 = call <vilib>:"Check if File or Folder Exists.vi"("path"=w515) -> ("file or folder exists?"=w516:bool, "dup path"=w517:path)  [unwired: 8 in, 1 out]
            n333 = call <vilib>:"Check if File or Folder Exists.vi"("path"=w518) -> ("file or folder exists?"=w521:bool, "dup path"=w522:path)  [unwired: 8 in, 1 out]
            n334 = Concatenate Strings("http://127.0.0.1:5000/openqq/send_friend_message?id=" ("字符串"), w533, "&content=!stop!" ("字符串")) -> (w529:string)
            n335 = case shown="真" w521 {
              tunnel: w522 -> [_ w537]
              frame False {
              }
              frame True {
                n336 = Delete(path (use dialog)=w537) -> ()  [unwired: 4 in, 3 out]
              }
            }
            n337 = case shown="真" w516 {
              tunnel: w517 -> [_ w538]
              frame False {
              }
              frame True {
                n338 = Delete(path (use dialog)=w538) -> ()  [unwired: 4 in, 3 out]
              }
            }
            n339 = call <vilib>:"OpenHandle.vi"() -> ("client handle out"=w525:T7)  [unwired: 14 in, 1 out]
            n340 = Text to UTF-8(11:w529) -> (3:w526:string)  [unwired: 2 in, 1 out]
            n341 = call <vilib>:"GET.vi"("client handle"=w525, "url"=w526) -> ("client handle out"=w524:T7, "error out"=w527:errorcluster)  [unwired: 10 in, 2 out]
            n342 = call <vilib>:"CloseHandle.vi"("client handle"=w524) -> ()  [unwired: 14 in, 1 out]
            n343 = call <vilib>:"Clear Errors.vi"("error in (no error)"=w527) -> ()  [unwired: 5 in, 2 out]
            n344 = call <vilib>:"General Error Handler.vi"() -> ()  [unwired: 11 in, 5 out]
          }
          frame #1 {
            w539 = "" ("接收者的QQ昵称或备注名")
            w540 = T5."Disabled and Grayed Out" ("禁用")
            n345 = property on="接收者的QQ昵称或备注名" class="Str"("DisabledEnum"=w540) -> ()  [unwired: 2 in, 2 out]
            n346 = property on="搜索ID按钮" class="Bool"("DisabledEnum"=w540) -> ()  [unwired: 2 in, 2 out]
            n347 = property on="确认发送实时日志" class="Bool (严格)"("DisabledEnum"=w540) -> ()  [unwired: 2 in, 2 out]
            n348 = property on="退出QQ号按钮" class="Bool"("DisabledEnum"=w540) -> ()  [unwired: 2 in, 2 out]
            n349 = property on="接收者的QQ昵称或备注名" class="Str"("Value"=w539) -> ()  [unwired: 2 in, 2 out]
            n350 = property on="接受者ID" class="Str"("Value"=w539) -> ()  [unwired: 2 in, 2 out]
          }
        }
      }
      event Panel Close? {
        n351 = event-data() -> ()  [unwired: 1 in, 4 out]
        n352 = event-data() -> ()  [unwired: 2 in, 1 out]
      }
      event "清扫速度确认": Value Change {
        n353 = event-data() -> ()  [unwired: 1 in, 6 out]
        n354 = formula code="Y=X*15+105;"("X"="清扫速度：") -> ("Y"=w542:dbl)
        n355 = Number To Decimal String(number=w542) -> (decimal integer string=w547:string)  [unwired: 1 in]
        n356 = Concatenate Strings("pwm" ("字符串"), w547) -> (w541:string)
        n357 = TCP Write(connection ID=w543, data in=w541) -> (connection ID out=w544:refnum<k5>, error out=w546:errorcluster)  [unwired: 2 in, 1 out]
        n358 = property on="清扫速度：" class="Str"("Value"=w541) -> ()  [unwired: 2 in, 2 out]
        n359 = call <vilib>:"Clear Errors.vi"("error in (no error)"=w546) -> ("error out"=w545:errorcluster)  [unwired: 5 in, 1 out]
        n360 = call <vilib>:"Simple Error Handler.vi"("error in (no error)"=w545) -> ()  [unwired: 4 in, 5 out]
      }
      event "清扫模式选择开关": Value Change {
        # "智能清扫为ON/真"
        n361 = event-data() -> ()  [unwired: 1 in, 6 out]
        n362 = case shown="真" "清扫模式选择开关" {
          tunnel: w551 -> [w554 w571]
          tunnel: [w553 w570] -> w550
          frame False {
            # "手动清扫模式"
            n363 = property on="连接状态" class="Bool (严格)"() -> ("Value"=w555:bool)  [unwired: 2 in, 2 out]
            n364 = case shown="假" w555 {
              tunnel: w554 -> [w556 w559]
              tunnel: [w556 w558] -> w553
              frame False {
                w557 = T5."Disabled and Grayed Out" ("禁用")
                n365 = property on="确认定时" class="Bool"("DisabledEnum"=w557) -> ()  [unwired: 2 in, 2 out]
                n366 = property on="清扫速度确认" class="Bool"("DisabledEnum"=w557) -> ()  [unwired: 2 in, 2 out]
                n367 = property on="清扫周期：" class="Ring (严格)"("DisabledEnum"=w557) -> ()  [unwired: 2 in, 2 out]
                n368 = property on="清扫速度：" class="Slide (严格)"("DisabledEnum"=w557) -> ()  [unwired: 2 in, 2 out]
              }
              frame True {
                w569 = T5."Enabled" ("禁用")
                n369 = property on="清扫速度：" class="Slide (严格)"() -> ("Value"=w560:i32)  [unwired: 2 in, 2 out]
                n370 = property on="确认定时" class="Bool"("DisabledEnum"=w569) -> ()  [unwired: 2 in, 2 out]
                n371 = property on="清扫速度确认" class="Bool"("DisabledEnum"=w569) -> ()  [unwired: 2 in, 2 out]
                n372 = property on="清扫周期：" class="Ring (严格)"("DisabledEnum"=w569) -> ()  [unwired: 2 in, 2 out]
                n373 = property on="清扫速度：" class="Slide (严格)"("DisabledEnum"=w569) -> ()  [unwired: 2 in, 2 out]
                n374 = formula code="Y=X*15+105;"("X"=w560) -> ("Y"=w561:dbl)
                n375 = property on="清扫周期：" class="Ring (严格)"() -> ("Value"=w568:dbl)  [unwired: 2 in, 2 out]
                n376 = property on="智能清扫模式确定按钮" class="Bool"("DisabledEnum"=T5."Disabled and Grayed Out" ("禁用")) -> ()  [unwired: 2 in, 2 out]
                n377 = Number To Decimal String(number=w561) -> (decimal integer string=w563:string)  [unwired: 1 in]
                n378 = property on="定时数" class="DigNum (严格)"("Value"=w568) -> ()  [unwired: 2 in, 2 out]
                n379 = Concatenate Strings("pwm" ("字符串"), w563) -> (w566:string)
                n380 = property on="清扫速度：" class="Str"("Value"=w566) -> ()  [unwired: 2 in, 2 out]
                n381 = TCP Write(connection ID=w559, data in=w566) -> (connection ID out=w558:refnum<k5>, error out=w564:errorcluster)  [unwired: 2 in, 1 out]
                n382 = call <vilib>:"Clear Errors.vi"("error in (no error)"=w564) -> ("error out"=w565:errorcluster)  [unwired: 5 in, 1 out]
                n383 = call <vilib>:"Simple Error Handler.vi"("error in (no error)"=w565) -> ()  [unwired: 4 in, 5 out]
              }
            }
          }
          frame True {
            # "智能清扫模式"
            n384 = property on="连接状态" class="Bool (严格)"() -> ("Value"=w572:bool)  [unwired: 2 in, 2 out]
            n385 = case shown="真" w572 {
              tunnel: w571 -> [w574 w576]
              tunnel: [w574 w575] -> w570
              frame False {
                n386 = property on="智能清扫模式确定按钮" class="Bool"("DisabledEnum"=T5."Disabled and Grayed Out" ("禁用")) -> ()  [unwired: 2 in, 2 out]
              }
              frame True {
                n387 = stacked-sequence {
                  tunnel: w576 -> [_ w588]
                  tunnel: [_ w587] -> w575
                  frame #0 {
                    n388 = flat-sequence {
                      frame #0 {
                        n389 = property on="当前城市" class="Str"() -> ("Value"=w578:string)  [unwired: 2 in, 2 out]
                        n390 = call "抓取天气查询.vi"("城市（市，县）"=w578) -> ("当前天气"=w577:string)
                        n391 = property on="天气：" class="Str"("Value"=w577) -> ()  [unwired: 2 in, 2 out]
                      }
                      frame #1 {
                        n392 = property on="天气：" class="Str"() -> ("Value"=w579:string)  [unwired: 2 in, 2 out]
                        n393 = Concatenate Strings("和风天气图标\\" ("字符串"), w579, ".png" ("字符串")) -> (w582:string)
                        n394 = call <vilib>:"Application Directory.vi"() -> ("Application Directory"=w581:path)
                        n395 = Build Path(base path=w581, name or relative path=w582) -> (appended path=w580:path)
                        n396 = call "显示图片.vi"("路径"=w580, "缩放因子"=1.1) -> ("二维图片"=w586:T2)  [unwired: 8 in]
                        n397 = property on="天气图标" class="Pict (严格)"("Value"=w586) -> ()  [unwired: 2 in, 2 out]
                      }
                    }
                  }
                  frame #1 {
                    w599 = T5."Disabled and Grayed Out" ("禁用")
                    n398 = property on="天气：" class="Str"() -> ("Value"=w596:string)  [unwired: 2 in, 2 out]
                    n399 = case shown="\"浮尘\", \"龙卷风\", \"强沙尘暴\", \"沙尘暴\", \"扬沙\"" w596 {
                      tunnel: [w600 w601 w602 w603 w604 w605] -> w589
                      frame "假", Default {
                        # "其他"
                        n400 = property on="其他类清扫速度：" class="Slide (严格)"() -> ("Value"=w600:i32)  [unwired: 2 in, 2 out]
                      }
                      frame "晴", "晴间多云" {
                        # "晴类"
                        n401 = property on="晴类清扫速度：" class="Slide (严格)"() -> ("Value"=w601:i32)  [unwired: 2 in, 2 out]
                      }
                      frame "薄雾", "多云", "少云", "雾", "阴", "霾" {
                        # "阴类"
                        n402 = property on="阴类清扫速度：" class="Slide (严格)"() -> ("Value"=w602:i32)  [unwired: 2 in, 2 out]
                      }
                      frame "暴雨", "大暴雨", "大雨", "极端降雨", "雷阵雨", "毛毛雨", "强雷阵雨", "强阵雨", "特大暴雨", "细雨", "小雨", "阵雨", "中雨" {
                        # "雨类"
                        n403 = property on="雨类清扫速度：" class="Slide (严格)"() -> ("Value"=w603:i32)  [unwired: 2 in, 2 out]
                      }
                      frame "暴雪", "大雪", "冻雨", "雷阵雨伴有冰雹", "小雪", "雨夹雪", "雨雪天气", "阵雪", "阵雨夹雪", "中雪" {
                        # "雪类"
                        n404 = property on="雪类清扫速度：" class="Slide (严格)"() -> ("Value"=w604:i32)  [unwired: 2 in, 2 out]
                      }
                      frame "浮尘", "龙卷风", "强沙尘暴", "沙尘暴", "扬沙" {
                        # "沙尘类"
                        n405 = property on="沙尘类清扫速度：" class="Slide (严格)"() -> ("Value"=w605:i32)  [unwired: 2 in, 2 out]
                      }
                    }
                    n406 = property on="天气：" class="Str"() -> ("Value"=w598:string)  [unwired: 2 in, 2 out]
                    n407 = formula code="Y=X*15+105;"("X"=w589) -> ("Y"=w595:dbl)
                    n408 = case shown="\"薄雾\", \"多云\", \"少云\", \"雾\", \"阴\", \"霾\"" w598 {
                      frame "假", Default {
                        n409 = property on="其他类清扫周期：" class="Ring (严格)"() -> ("Value"=w606:dbl)  [unwired: 2 in, 2 out]
                        n410 = property on="定时数" class="DigNum (严格)"("Value"=w606) -> ()  [unwired: 2 in, 2 out]
                      }
                      frame "晴", "晴间多云" {
                        # "晴类"
                        n411 = property on="晴类清扫周期：" class="Ring (严格)"() -> ("Value"=w607:dbl)  [unwired: 2 in, 2 out]
                        n412 = property on="定时数" class="DigNum (严格)"("Value"=w607) -> ()  [unwired: 2 in, 2 out]
                      }
                      frame "薄雾", "多云", "少云", "雾", "阴", "霾" {
                        # "阴类"
                        n413 = property on="阴类清扫周期：" class="Ring (严格)"() -> ("Value"=w608:dbl)  [unwired: 2 in, 2 out]
                        n414 = property on="定时数" class="DigNum (严格)"("Value"=w608) -> ()  [unwired: 2 in, 2 out]
                      }
                      frame "暴雨", "大暴雨", "大雨", "极端降雨", "雷阵雨", "毛毛雨", "强雷阵雨", "强阵雨", "特大暴雨", "细雨", "小雨", "阵雨", "中雨" {
                        # "雨类"
                        n415 = property on="雨类清扫周期：" class="Ring (严格)"() -> ("Value"=w609:dbl)  [unwired: 2 in, 2 out]
                        n416 = property on="定时数" class="DigNum (严格)"("Value"=w609) -> ()  [unwired: 2 in, 2 out]
                      }
                      frame "暴雪", "大雪", "冻雨", "雷阵雨伴有冰雹", "小雪", "雨夹雪", "雨雪天气", "阵雪", "阵雨夹雪", "中雪" {
                        # "雪类"
                        n417 = property on="雪类清扫周期：" class="Ring (严格)"() -> ("Value"=w610:dbl)  [unwired: 2 in, 2 out]
                        n418 = property on="定时数" class="DigNum (严格)"("Value"=w610) -> ()  [unwired: 2 in, 2 out]
                      }
                      frame "浮尘", "龙卷风", "强沙尘暴", "沙尘暴", "扬沙" {
                        # "沙尘类"
                        n419 = property on="沙尘类清扫周期：" class="Ring (严格)"() -> ("Value"=w611:dbl)  [unwired: 2 in, 2 out]
                        n420 = property on="定时数" class="DigNum (严格)"("Value"=w611) -> ()  [unwired: 2 in, 2 out]
                      }
                    }
                    n421 = property on="确认定时" class="Bool"("DisabledEnum"=w599) -> ()  [unwired: 2 in, 2 out]
                    n422 = property on="清扫速度确认" class="Bool"("DisabledEnum"=w599) -> ()  [unwired: 2 in, 2 out]
                    n423 = property on="清扫周期：" class="Ring (严格)"("DisabledEnum"=w599) -> ()  [unwired: 2 in, 2 out]
                    n424 = property on="清扫速度：" class="Slide (严格)"("DisabledEnum"=w599) -> ()  [unwired: 2 in, 2 out]
                    n425 = Number To Decimal String(number=w595) -> (decimal integer string=w593:string)  [unwired: 1 in]
                    n426 = Concatenate Strings("pwm" ("字符串"), w593) -> (w590:string)
                    n427 = property on="智能清扫模式确定按钮" class="Bool"("DisabledEnum"=T5."Enabled" ("禁用")) -> ()  [unwired: 2 in, 2 out]
                    n428 = property on="清扫速度：" class="Str"("Value"=w590) -> ()  [unwired: 2 in, 2 out]
                    n429 = TCP Write(connection ID=w588, data in=w590) -> (connection ID out=w587:refnum<k5>, error out=w592:errorcluster)  [unwired: 2 in, 1 out]
                    n430 = call <vilib>:"Clear Errors.vi"("error in (no error)"=w592) -> ("error out"=w591:errorcluster)  [unwired: 5 in, 1 out]
                    n431 = call <vilib>:"Simple Error Handler.vi"("error in (no error)"=w591) -> ()  [unwired: 4 in, 5 out]
                  }
                }
              }
            }
          }
        }
      }
      event "发送按钮": Value Change {
        n432 = event-data() -> ()  [unwired: 1 in, 6 out]
        n433 = TCP Write(connection ID=w616, data in="待发送数据", 9:500 ("超时毫秒(25000)")) -> (connection ID out=w615:refnum<k5>, error out=w614:errorcluster)  [unwired: 1 in, 1 out]
      }
      event "断开连接": Value Change {
        w617 = "未运行" ("清扫速度：")
        w619 = T5."Disabled and Grayed Out" ("禁用")
        n434 = event-data() -> ()  [unwired: 1 in, 6 out]
        n435 = TCP Close Connection(connection ID=w621) -> (connection ID out=w618:refnum<k5>, error out=→"错误输出 2":errorcluster)  [unwired: 2 in]
        n436 = local write "连接状态"(FALSE ("连接状态")) -> ()
        n437 = local write "控制器IP："("" ("控制器IP：")) -> ()
        n438 = property on="连接控制器" class="Bool"("DisabledEnum"=T5."Enabled" ("禁用")) -> ()  [unwired: 2 in, 2 out]
        n439 = property on="断开连接" class="Bool"("DisabledEnum"=w619) -> ()  [unwired: 2 in, 2 out]
        n440 = property on="清扫速度确认" class="Bool"("DisabledEnum"=w619) -> ()  [unwired: 2 in, 2 out]
        n441 = property on="确认定时" class="Bool"("DisabledEnum"=w619) -> ()  [unwired: 2 in, 2 out]
        n442 = property on="开灯" class="Bool"("DisabledEnum"=w619) -> ()  [unwired: 2 in, 2 out]
        n443 = property on="发送按钮" class="Bool"("DisabledEnum"=w619) -> ()  [unwired: 2 in, 2 out]
        n444 = property on="清扫周期：" class="Str"("Value"=w617) -> ()  [unwired: 2 in, 2 out]
        n445 = property on="清扫速度：" class="Str"("Value"=w617) -> ()  [unwired: 2 in, 2 out]
      }
      event "查看项目主页按钮": Value Change {
        n446 = event-data() -> ()  [unwired: 1 in, 6 out]
        n447 = call <vilib>:"System Exec.vi"("run minimized? (F)"=TRUE, "command line"="CMD /C start  https://github.com/skkkyoyo/Controller-of-solar-roof-cleaning-robot") -> ()  [unwired: 6 in, 4 out]
      }
      event "清空接收区按钮": Value Change {
        n448 = event-data() -> ()  [unwired: 1 in, 6 out]
        n449 = property on="数据接收显示" class="Str"("Value"="下列为接收到的数据..." ("数据接收显示")) -> ()  [unwired: 2 in, 2 out]
      }
      event "确认定时": Value Change {
        n450 = event-data() -> ()  [unwired: 1 in, 6 out]
        n451 = flat-sequence {
          frame #0 {
            n452 = property on="清扫周期：" class="Ring (严格)"() -> ("Value"=w631:dbl)  [unwired: 2 in, 2 out]
            n453 = property on="定时数" class="DigNum (严格)"("Value"=w631) -> ()  [unwired: 2 in, 2 out]
          }
          frame #1 {
            n454 = property on="定时数" class="DigNum (严格)"() -> ("Value"=w633:dbl)  [unwired: 2 in, 2 out]
            n455 = Number To Fractional String(number=w633, precision (6)=i16 1 ("精度(6)")) -> (F-format string=w635:string)  [unwired: 2 in]
            n456 = Concatenate Strings(w635, "小时" ("字符串")) -> (w636:string)
            n457 = property on="清扫周期：" class="Str"("Value"=w636) -> ()  [unwired: 2 in, 2 out]
          }
        }
      }
      event "智能清扫模式确定按钮": Value Change {
        n458 = event-data() -> ()  [unwired: 1 in, 6 out]
        n459 = flat-sequence {
          tunnel: w639 -> [w641]
          tunnel: [w640] -> w637
          tunnel: [w697] -> w638
          tunnel: w637 -> [w697]
          frame #0 {
            n460 = property on="天气：" class="Str"() -> ("Value"=w649:string)  [unwired: 2 in, 2 out]
            n461 = case shown="\"假\", 默认" w649 {
              tunnel: [w650 w651 w652 w653 w654 w655] -> w642
              frame "假", Default {
                # "其他"
                n462 = property on="其他类清扫速度：" class="Slide (严格)"() -> ("Value"=w650:i32)  [unwired: 2 in, 2 out]
              }
              frame "晴", "晴间多云" {
                # "晴类"
                n463 = property on="晴类清扫速度：" class="Slide (严格)"() -> ("Value"=w651:i32)  [unwired: 2 in, 2 out]
              }
              frame "薄雾", "多云", "少云", "雾", "阴", "霾" {
                # "阴类"
                n464 = property on="阴类清扫速度：" class="Slide (严格)"() -> ("Value"=w652:i32)  [unwired: 2 in, 2 out]
              }
              frame "暴雨", "大暴雨", "大雨", "极端降雨", "雷阵雨", "毛毛雨", "强雷阵雨", "强阵雨", "特大暴雨", "细雨", "小雨", "阵雨", "中雨" {
                # "雨类"
                n465 = property on="雨类清扫速度：" class="Slide (严格)"() -> ("Value"=w653:i32)  [unwired: 2 in, 2 out]
              }
              frame "暴雪", "大雪", "冻雨", "雷阵雨伴有冰雹", "小雪", "雨夹雪", "雨雪天气", "阵雪", "阵雨夹雪", "中雪" {
                # "雪类"
                n466 = property on="雪类清扫速度：" class="Slide (严格)"() -> ("Value"=w654:i32)  [unwired: 2 in, 2 out]
              }
              frame "浮尘", "龙卷风", "强沙尘暴", "沙尘暴", "扬沙" {
                # "沙尘类"
                n467 = property on="沙尘类清扫速度：" class="Slide (严格)"() -> ("Value"=w655:i32)  [unwired: 2 in, 2 out]
              }
            }
            n468 = flat-sequence {
              frame #0 {
                # "运行周期确认"
                n469 = property on="天气：" class="Str"() -> ("Value"=w656:string)  [unwired: 2 in, 2 out]
                n470 = case shown="\"浮尘\", \"龙卷风\", \"强沙尘暴\", \"沙尘暴\", \"扬沙\"" w656 {
                  frame "假", Default {
                    n471 = property on="其他类清扫周期：" class="Ring (严格)"() -> ("Value"=w657:dbl)  [unwired: 2 in, 2 out]
                    n472 = property on="定时数" class="DigNum (严格)"("Value"=w657) -> ()  [unwired: 2 in, 2 out]
                  }
                  frame "晴", "晴间多云" {
                    # "晴类"
                    n473 = property on="晴类清扫周期：" class="Ring (严格)"() -> ("Value"=w658:dbl)  [unwired: 2 in, 2 out]
                    n474 = property on="定时数" class="DigNum (严格)"("Value"=w658) -> ()  [unwired: 2 in, 2 out]
                  }
                  frame "薄雾", "多云", "少云", "雾", "阴", "霾" {
                    # "阴类"
                    n475 = property on="阴类清扫周期：" class="Ring (严格)"() -> ("Value"=w659:dbl)  [unwired: 2 in, 2 out]
                    n476 = property on="定时数" class="DigNum (严格)"("Value"=w659) -> ()  [unwired: 2 in, 2 out]
                  }
                  frame "暴雨", "大暴雨", "大雨", "极端降雨", "雷阵雨", "毛毛雨", "强雷阵雨", "强阵雨", "特大暴雨", "细雨", "小雨", "阵雨", "中雨" {
                    # "雨类"
                    n477 = property on="雨类清扫周期：" class="Ring (严格)"() -> ("Value"=w660:dbl)  [unwired: 2 in, 2 out]
                    n478 = property on="定时数" class="DigNum (严格)"("Value"=w660) -> ()  [unwired: 2 in, 2 out]
                  }
                  frame "暴雪", "大雪", "冻雨", "雷阵雨伴有冰雹", "小雪", "雨夹雪", "雨雪天气", "阵雪", "阵雨夹雪", "中雪" {
                    # "雪类"
                    n479 = property on="雪类清扫周期：" class="Ring (严格)"() -> ("Value"=w661:dbl)  [unwired: 2 in, 2 out]
                    n480 = property on="定时数" class="DigNum (严格)"("Value"=w661) -> ()  [unwired: 2 in, 2 out]
                  }
                  frame "浮尘", "龙卷风", "强沙尘暴", "沙尘暴", "扬沙" {
                    # "沙尘类"
                    n481 = property on="沙尘类清扫周期：" class="Ring (严格)"() -> ("Value"=w662:dbl)  [unwired: 2 in, 2 out]
                    n482 = property on="定时数" class="DigNum (严格)"("Value"=w662) -> ()  [unwired: 2 in, 2 out]
                  }
                }
              }
              frame #1 {
                n483 = property on="定时数" class="DigNum (严格)"() -> ("Value"=w666:dbl)  [unwired: 2 in, 2 out]
                n484 = Number To Decimal String(number=w666) -> (decimal integer string=w664:string)  [unwired: 1 in]
                n485 = Concatenate Strings(w664, "小时" ("字符串")) -> (w663:string)
                n486 = property on="清扫周期：" class="Str"("Value"=w663) -> ()  [unwired: 2 in, 2 out]
              }
            }
            n487 = formula code="Y=X*15+149;"("X"=w642) -> ("Y"=w648:dbl)
            n488 = Number To Decimal String(number=w648) -> (decimal integer string=w646:string)  [unwired: 1 in]
            n489 = Concatenate Strings("pwm" ("字符串"), w646) -> (w643:string)
            n490 = property on="清扫速度：" class="Str"("Value"=w643) -> ()  [unwired: 2 in, 2 out]
            n491 = TCP Write(connection ID=w641, data in=w643) -> (connection ID out=w640:refnum<k5>, error out=w645:errorcluster)  [unwired: 2 in, 1 out]
            n492 = call <vilib>:"Clear Errors.vi"("error in (no error)"=w645) -> ("error out"=w644:errorcluster)  [unwired: 5 in, 1 out]
            n493 = call <vilib>:"Simple Error Handler.vi"("error in (no error)"=w644) -> ()  [unwired: 4 in, 5 out]
          }
          frame #1 {
            w680 = 0 ("禁用的索引 (列)")
            w695 = 1 ("禁用的索引 (列)")
            n494 = property on="沙尘类清扫周期：" class="Ring (严格)"() -> ("Value"=w678:dbl)  [unwired: 2 in, 2 out]
            n495 = property on="雪类清扫周期：" class="Ring (严格)"() -> ("Value"=w676:dbl)  [unwired: 2 in, 2 out]
            n496 = property on="雨类清扫周期：" class="Ring (严格)"() -> ("Value"=w674:dbl)  [unwired: 2 in, 2 out]
            n497 = property on="其他类清扫周期：" class="Ring (严格)"() -> ("Value"=w681:dbl)  [unwired: 2 in, 2 out]
            n498 = property on="阴类清扫周期：" class="Ring (严格)"() -> ("Value"=w672:dbl)  [unwired: 2 in, 2 out]
            n499 = property on="晴类清扫周期：" class="Ring (严格)"() -> ("Value"=w668:dbl)  [unwired: 2 in, 2 out]
            n500 = property on="清扫模式记录数组" class="Arr (严格)"() -> ("Value"=w667:dbl[][])  [unwired: 2 in, 2 out]
            n501 = Replace Array Subset(array=w667, new element #1=w668, index (row) #1=0 ("索引 (行)"), index (col) #1=w680, new element #2=w672, index (row) #2=1 ("索引 (行)"), index (col) #2=w680, new element #3=w674, index (row) #3=2 ("索引 (行)"), index (col) #3=w680, new element #4=w676, index (row) #4=3 ("索引 (行)"), index (col) #4=w680, new element #5=w678, index (row) #5=4 ("索引 (行)"), index (col) #5=w680, new element #6=w681, index (row) #6=5 ("索引 (行)"), index (col) #6=w680) -> (w669:dbl[][])
            n502 = property on="雪类清扫速度：" class="Slide (严格)"() -> ("Value"=w691:i32)  [unwired: 2 in, 2 out]
            n503 = property on="晴类清扫速度：" class="Slide (严格)"() -> ("Value"=w685:i32)  [unwired: 2 in, 2 out]
            n504 = property on="阴类清扫速度：" class="Slide (严格)"() -> ("Value"=w687:i32)  [unwired: 2 in, 2 out]
            n505 = property on="雨类清扫速度：" class="Slide (严格)"() -> ("Value"=w689:i32)  [unwired: 2 in, 2 out]
            n506 = property on="沙尘类清扫速度：" class="Slide (严格)"() -> ("Value"=w693:i32)  [unwired: 2 in, 2 out]
            n507 = property on="其他类清扫速度：" class="Slide (严格)"() -> ("Value"=w696:i32)  [unwired: 2 in, 2 out]
            n508 = property on="清扫模式记录数组" class="Arr (严格)"("Value"=w669) -> ()  [unwired: 2 in, 2 out]
            n509 = property on="清扫模式记录数组" class="Arr (严格)"() -> ("Value"=w682:dbl[][])  [unwired: 2 in, 2 out]
            n510 = Replace Array Subset(array=w682, new element #1=w685, index (row) #1=0 ("索引 (行)"), index (col) #1=w695, new element #2=w687, index (row) #2=1 ("索引 (行)"), index (col) #2=w695, new element #3=w689, index (row) #3=2 ("索引 (行)"), index (col) #3=w695, new element #4=w691, index (row) #4=3 ("索引 (行)"), index (col) #4=w695, new element #5=w693, index (row) #5=4 ("索引 (行)"), index (col) #5=w695, new element #6=w696, index (row) #6=5 ("索引 (行)"), index (col) #6=w695) -> (w683:dbl[][])
            n511 = property on="清扫模式记录数组" class="Arr (严格)"("Value"=w683) -> ()  [unwired: 2 in, 2 out]
          }
        }
      }
      event "开灯": Value Change {
        n512 = event-data() -> ()  [unwired: 1 in, 6 out]
        n513 = flat-sequence {
          tunnel: [w706] -> w702
          tunnel: [w704] -> w701
          tunnel: w700 -> [w703]
          tunnel: [w709] -> w699
          tunnel: w702 -> [w710]
          tunnel: w701 -> [w712]
          tunnel: [w711] -> w698
          frame #0 {
            n514 = TCP Write(connection ID=w703, data in="ledon" ("数据输入")) -> (connection ID out=w704:refnum<k5>, error out=w706:errorcluster)  [unwired: 2 in, 1 out]
            n515 = Wait (ms)(milliseconds to wait=u32 1000 ("等待时间（毫秒）")) -> ()  [unwired: 1 out]
          }
          frame #1 {
            n516 = TCP Write(connection ID=w712, data in="ledoff" ("数据输入"), error in (no error)=w710) -> (connection ID out=w711:refnum<k5>, error out=w709:errorcluster)  [unwired: 1 in, 1 out]
          }
        }
      }
      event "一直开灯": Value Change {
        n517 = event-data() -> ()  [unwired: 1 in, 6 out]
        n518 = TCP Write(connection ID=w715, data in="ledon" ("数据输入")) -> (connection ID out=w714:refnum<k5>, error out=w713:errorcluster)  [unwired: 2 in, 1 out]
      }
    }
    n519 = property on="webqq好友" class="Str" props=["Value"]() -> ()  [unwired: 2 in, 3 out]
    n520 = property on="接收者的QQ昵称或备注名" class="Str" props=["Value"]() -> ()  [unwired: 2 in, 3 out]
    n521 = property on="清扫命令发出标志" class="Bool (严格)"() -> ("Value"=w256:bool)  [unwired: 2 in, 2 out]
    n522 = case shown="真" w256 {
      tunnel: w259 -> [w333 w339]
      tunnel: [w333 w338] -> w254
      tunnel: w258 -> [w334 w337]
      tunnel: [w334 w336] -> w257
      frame False {
      }
      frame True {
        n523 = flat-sequence {
          tunnel: w339 -> [w344]
          tunnel: w337 -> [w342]
          tunnel: [w341] -> w336
          tunnel: [w343] -> w335
          tunnel: [w348] -> w338
          tunnel: w335 -> [w348]
          frame #0 {
            n524 = TCP Write(connection ID=w344, data in="clean" ("数据输入"), error in (no error)=w342, 9:500 ("超时毫秒(25000)")) -> (connection ID out=w343:refnum<k5>, error out=w341:errorcluster)  [unwired: 1 out]
            n525 = Wait (ms)(milliseconds to wait=u32 100 ("等待时间（毫秒）")) -> ()  [unwired: 1 out]
          }
          frame #1 {
            n526 = property on="清扫命令发出标志" class="Bool (严格)"("Value"=FALSE ("清扫命令发出")) -> ()  [unwired: 2 in, 2 out]
          }
        }
      }
    }
    n527 = case shown="假" "刷新标志" {
      tunnel: w254 -> [w285 w303]
      tunnel: [w285 w301] -> w253
      frame False {
        n528 = disable-structure shown="禁用" {
          frame Disabled {
            n529 = call "获取时间.vi"() -> ("当前秒"=w292:string)  [unwired: 8 in, 3 out]
            n530 = Decimal String To Number(string=w292) -> (number=w291:i32)  [unwired: 2 in, 1 out]
            n531 = Quotient & Remainder(x=w291, y=5) -> (x-y*floor(x/y)=w289:i32)  [unwired: 1 out]
            n532 = Equal?(x=w289, y=0 ("x-y*floor(x/y)")) -> (x = y?=w287:bool)
            n533 = case shown="真" w287 {
              tunnel: [w293 w299] -> w286
              tunnel: [w293 w298] -> _
              frame False {
              }
              frame True {
                # "心跳认证"
                n534 = TCP Write(connection ID=w299, data in="heartbeat " ("数据输入")) -> (connection ID out=w298:refnum<k5>, error out=w294:errorcluster)  [unwired: 2 in, 1 out]
                n535 = call <vilib>:"Clear Errors.vi"("error in (no error)"=w294) -> ("error out"=w295:errorcluster)  [unwired: 5 in, 1 out]
                n536 = call <vilib>:"Simple Error Handler.vi"("error in (no error)"=w295) -> ()  [unwired: 4 in, 5 out]
                "心跳认证标志" <- TRUE ("心跳认证标志")
              }
            }
          }
          frame Enabled {
          }
        }
      }
      frame True {
        n537 = property on="天气：" class="Str"() -> ("Value"=w305:string)  [unwired: 2 in, 2 out]
        n538 = case shown="\"浮尘\", \"龙卷风\", \"强沙尘暴\", \"沙尘暴\", \"扬沙\"" w305 {
          frame "假", Default {
            # "其他"
            n539 = property on="清扫模式记录数组" class="Arr (严格)"() -> ("Value"=w312:dbl[][])  [unwired: 2 in, 2 out]
            n540 = Index Array(array=w312, index (row)=5 ("索引 (行)"), index (col)=1 ("禁用的索引 (列)")) -> (element=w309:dbl)
            n541 = property on="刷新时的PWM数值" class="DigNum (严格)"("Value"=w309) -> ()  [unwired: 2 in, 2 out]
          }
          frame "晴", "晴间多云" {
            # "晴类"
            n542 = property on="清扫模式记录数组" class="Arr (严格)"() -> ("Value"=w314:dbl[][])  [unwired: 2 in, 2 out]
            n543 = Index Array(array=w314, index (row)=0 ("索引 (行)"), index (col)=1 ("禁用的索引 (列)")) -> (element=w313:dbl)
            n544 = property on="刷新时的PWM数值" class="DigNum (严格)"("Value"=w313) -> ()  [unwired: 2 in, 2 out]
          }
          frame "薄雾", "多云", "少云", "雾", "阴", "霾" {
            # "阴类"
            n545 = property on="清扫模式记录数组" class="Arr (严格)"() -> ("Value"=w320:dbl[][])  [unwired: 2 in, 2 out]
            n546 = Index Array(array=w320, index (row)=1 ("索引 (行)"), index (col)=1 ("禁用的索引 (列)")) -> (element=w317:dbl)
            n547 = property on="刷新时的PWM数值" class="DigNum (严格)"("Value"=w317) -> ()  [unwired: 2 in, 2 out]
          }
          frame "暴雨", "大暴雨", "大雨", "极端降雨", "雷阵雨", "毛毛雨", "强雷阵雨", "强阵雨", "特大暴雨", "细雨", "小雨", "阵雨", "中雨" {
            # "雨类"
            n548 = property on="清扫模式记录数组" class="Arr (严格)"() -> ("Value"=w324:dbl[][])  [unwired: 2 in, 2 out]
            n549 = Index Array(array=w324, index (row)=2 ("索引 (行)"), index (col)=1 ("禁用的索引 (列)")) -> (element=w321:dbl)
            n550 = property on="刷新时的PWM数值" class="DigNum (严格)"("Value"=w321) -> ()  [unwired: 2 in, 2 out]
          }
          frame "暴雪", "大雪", "冻雨", "雷阵雨伴有冰雹", "小雪", "雨夹雪", "雨雪天气", "阵雪", "阵雨夹雪", "中雪" {
            # "雪类"
            n551 = property on="清扫模式记录数组" class="Arr (严格)"() -> ("Value"=w328:dbl[][])  [unwired: 2 in, 2 out]
            n552 = Index Array(array=w328, index (row)=3 ("索引 (行)"), index (col)=1 ("禁用的索引 (列)")) -> (element=w325:dbl)
            n553 = property on="刷新时的PWM数值" class="DigNum (严格)"("Value"=w325) -> ()  [unwired: 2 in, 2 out]
          }
          frame "浮尘", "龙卷风", "强沙尘暴", "沙尘暴", "扬沙" {
            # "沙尘类"
            n554 = property on="清扫模式记录数组" class="Arr (严格)"() -> ("Value"=w332:dbl[][])  [unwired: 2 in, 2 out]
            n555 = Index Array(array=w332, index (row)=4 ("索引 (行)"), index (col)=1 ("禁用的索引 (列)")) -> (element=w330:dbl)
            n556 = property on="刷新时的PWM数值" class="DigNum (严格)"("Value"=w330) -> ()  [unwired: 2 in, 2 out]
          }
        }
        n557 = property on="刷新标志" class="Bool (严格)"("Value"=FALSE ("刷新标志")) -> ()  [unwired: 2 in, 2 out]
        n558 = formula code="Y=X*15+105;"("X"="刷新时的PWM数值") -> ("Y"=w306:dbl)
        n559 = Number To Decimal String(number=w306) -> (decimal integer string=w308:string)  [unwired: 1 in]
        n560 = Concatenate Strings("pwm" ("字符串"), w308) -> (w304:string)
        n561 = property on="清扫速度：" class="Str"("Value"=w304) -> ()  [unwired: 2 in, 2 out]
        n562 = TCP Write(connection ID=w303, data in=w304) -> (connection ID out=w301:refnum<k5>)  [unwired: 2 in, 2 out]
      }
    }
    n563 = TCP Read(connection ID=w253, bytes to read=512, error in (no error)=w257, 9:50) -> (connection ID out=w245:refnum<k5>, data out=w263:string, error out=w252:errorcluster)  [unwired: 1 in]
    "错误输出" <- w252
    n564 = String Length(string=w263) -> (length=w261:i32)
    n565 = Greater Than 0?(x=w261) -> (x > 0?=w260:bool)
    n566 = case shown="真" w260 {
      tunnel: w263 -> [_ w351]
      frame False {
      }
      frame True {
        n567 = property on="数据接收显示" class="Str"() -> ("Value"=w358:string)  [unwired: 2 in, 2 out]
        n568 = Concatenate Strings(w358, "\r", w351) -> (w356:string)
        "数据接收显示" <- w356
        n569 = property on="待发送数据" class="Str"("Value"="" ("待发送数据")) -> ()  [unwired: 2 in, 2 out]
        n570 = String Length(string=w356) -> (length=w355:i32)
        n571 = property on="QQ状态" class="Bool (严格)"() -> ("Value"=w353:bool)  [unwired: 2 in, 2 out]
        n572 = String Length(string=w351) -> (length=w350:i32)
        n573 = property on="数据接收显示" class="Str"("Text.Scroll Position"=w355) -> ()  [unwired: 2 in, 2 out]
        n574 = Greater Than 0?(x=w350) -> (x > 0?=w349:bool)
        n575 = Compound Arithmetic op=AND ("复合运算")(w353, "确认发送实时日志", w349) -> (w354:bool)
        n576 = case shown="真" w354 {
          tunnel: w351 -> [_ w361]
          frame False {
          }
          frame True {
            # "QQ实时日志发送"
            n577 = property on="接受者ID" class="Str"() -> ("Value"=w365:string)  [unwired: 2 in, 2 out]
            n578 = call "获取时间.vi"() -> ("当前时间"=w362:string, "当前日期"=w364:string)  [unwired: 8 in, 2 out]
            n579 = Concatenate Strings("http://127.0.0.1:5000/openqq/send_friend_message?id=" ("字符串"), w365, "&content=" ("字符串"), w364, "  " ("字符串"), w362, "  " ("字符串"), w361) -> (w368:string)
            n580 = call <vilib>:"OpenHandle.vi"() -> ("client handle out"=w373:T7)  [unwired: 14 in, 1 out]
            n581 = Text to UTF-8(11:w368) -> (3:w370:string)  [unwired: 2 in, 1 out]
            n582 = call <vilib>:"GET.vi"("client handle"=w373, "url"=w370) -> ("client handle out"=w372:T7, "body"=w371:string, "error out"=w367:errorcluster)  [unwired: 10 in, 1 out]
            n583 = call <vilib>:"Clear Errors.vi"("error in (no error)"=w367) -> ("error out"=w366:errorcluster)  [unwired: 5 in, 1 out]
            n584 = call <vilib>:"CloseHandle.vi"("client handle"=w372) -> ()  [unwired: 14 in, 1 out]
            n585 = call <vilib>:"General Error Handler.vi"("error in (no error)"=w366) -> ()  [unwired: 10 in, 5 out]
            n586 = UTF-8 to Text(11:w371) -> (3:→"发送返回值":string)  [unwired: 2 in, 1 out]
          }
        }
      }
    }
    n587 = Unbundle(w252) -> ("code"=w249:i32)  [unwired: 2 out]
    n588 = Wait (ms)(milliseconds to wait=u32 50 ("等待时间（毫秒）")) -> ()  [unwired: 1 out]
    n589 = Equal?(x=66, y=w249) -> (x = y?=w248:bool)
    n590 = Equal?(x=w249, y=63) -> (x = y?=w247:bool)
    n591 = Or(x=w248, y=w247) -> (x .or. y?=w246:bool)
    n592 = case shown="真" w246 {
      tunnel: w245 -> [w269 w271]
      tunnel: [w269 w270] -> w244
      frame False {
      }
      frame True {
        n593 = One Button Dialog(message="链接似乎被中断" ("消息"), button name ("OK")="我已了解" ("按钮名称（“确定”）")) -> (true=w272:bool)
        n594 = case shown="真" w272 {
          tunnel: w271 -> [w275 w280]
          tunnel: [w275 w279] -> w270
          frame False {
          }
          frame True {
            w276 = "未运行" ("清扫速度：")
            w284 = T5."Disabled and Grayed Out" ("禁用")
            n595 = TCP Close Connection(connection ID=w280) -> (connection ID out=w279:refnum<k5>, error out=w277:errorcluster)  [unwired: 2 in]
            n596 = local write "控制器IP："("" ("控制器IP：")) -> ()
            n597 = local write "连接状态"(FALSE ("连接状态")) -> ()
            n598 = property on="清扫周期：" class="Str"("Value"=w276) -> ()  [unwired: 2 in, 2 out]
            n599 = property on="连接控制器" class="Bool"("DisabledEnum"=T5."Enabled" ("禁用")) -> ()  [unwired: 2 in, 2 out]
            n600 = call <vilib>:"Clear Errors.vi"("error in (no error)"=w277) -> ("error out"=w278:errorcluster)  [unwired: 5 in, 1 out]
            n601 = property on="清扫速度：" class="Str"("Value"=w276) -> ()  [unwired: 2 in, 2 out]
            n602 = call <vilib>:"Simple Error Handler.vi"("error in (no error)"=w278) -> ()  [unwired: 4 in, 5 out]
            n603 = property on="断开连接" class="Bool"("DisabledEnum"=w284) -> ()  [unwired: 2 in, 2 out]
            n604 = property on="清扫速度确认" class="Bool"("DisabledEnum"=w284) -> ()  [unwired: 2 in, 2 out]
            n605 = property on="确认定时" class="Bool"("DisabledEnum"=w284) -> ()  [unwired: 2 in, 2 out]
            n606 = property on="开灯" class="Bool"("DisabledEnum"=w284) -> ()  [unwired: 2 in, 2 out]
            n607 = property on="发送按钮" class="Bool"("DisabledEnum"=w284) -> ()  [unwired: 2 in, 2 out]
          }
        }
      }
    }
  }
  n608 = while {
    stop <- FALSE stop-if-true
    n609 = property on="正在加载标志" class="Bool (严格)"() -> ("Value"=w717:bool)  [unwired: 2 in, 2 out]
    n610 = case shown="真" w717 {
      frame False {
        n611 = property on="QQ状态" class="Bool (严格)"() -> ("Value"=w719:bool)  [unwired: 2 in, 2 out]
        n612 = case shown="真" w719 {
          frame False {
            n613 = call <vilib>:"Application Directory.vi"() -> ("Application Directory"=w724:path)
            n614 = Build Path(base path=w724, name or relative path="Mojo-StrawberryPerl\\tmp\\黑白QQ.png" ("名称或相对路径")) -> (appended path=w723:path)
            n615 = call <vilib>:"Read PNG File.vi"("path to PNG file"=w723) -> ("error out"=w721:errorcluster, "image data"=w726:T8)  [unwired: 8 in, 1 out]
            n616 = call <vilib>:"Draw Flattened Pixmap.vi"("image data"=w726) -> ("new picture"=w720:picture)  [unwired: 8 in]
            n617 = property on="QQ登录二维码" class="Pict"("Value"=w720) -> ()  [unwired: 2 in, 2 out]
            n618 = call <vilib>:"Clear Errors.vi"("error in (no error)"=w721) -> ("error out"=w722:errorcluster)  [unwired: 5 in, 1 out]
            n619 = call <vilib>:"General Error Handler.vi"("error in (no error)"=w722) -> ()  [unwired: 10 in, 5 out]
          }
          frame True {
            n620 = call <vilib>:"Application Directory.vi"() -> ("Application Directory"=w731:path)
            n621 = Build Path(base path=w731, name or relative path="Mojo-StrawberryPerl\\tmp\\彩色QQ.png" ("名称或相对路径")) -> (appended path=w730:path)
            n622 = call <vilib>:"Read PNG File.vi"("path to PNG file"=w730) -> ("error out"=w728:errorcluster, "image data"=w733:T8)  [unwired: 8 in, 1 out]
            n623 = call <vilib>:"Draw Flattened Pixmap.vi"("image data"=w733) -> ("new picture"=w727:picture)  [unwired: 8 in]
            n624 = property on="QQ登录二维码" class="Pict"("Value"=w727) -> ()  [unwired: 2 in, 2 out]
            n625 = call <vilib>:"Clear Errors.vi"("error in (no error)"=w728) -> ("error out"=w729:errorcluster)  [unwired: 5 in, 1 out]
            n626 = call <vilib>:"General Error Handler.vi"("error in (no error)"=w729) -> ()  [unwired: 10 in, 5 out]
          }
        }
      }
      frame True {
        n627 = call <vilib>:"Application Directory.vi"() -> ("Application Directory"=w737:path)
        n628 = Concatenate Strings("http://127.0.0.1:5000/openqq/get_friend_info" ("字符串")) -> (w749:string)
        n629 = Build Path(base path=w737, name or relative path="Mojo-StrawberryPerl\\tmp\\webqq.png" ("名称或相对路径")) -> (appended path=w736:path)
        "QQ二维码路径" <- w736
        n630 = call <vilib>:"Read PNG File.vi"("path to PNG file"=w736) -> ("error out"=w734:errorcluster, "image data"=w740:T8)  [unwired: 8 in, 1 out]
        n631 = call <vilib>:"OpenHandle.vi"() -> ("client handle out"=w744:T7)  [unwired: 14 in, 1 out]
        n632 = Text to UTF-8(11:w749) -> (3:w747:string)  [unwired: 2 in, 1 out]
        n633 = call <vilib>:"GET.vi"("client handle"=w744, "url"=w747) -> ("client handle out"=w745:T7, "body"=w746:string, "error out"=w750:errorcluster)  [unwired: 10 in, 1 out]
        n634 = call <vilib>:"Clear Errors.vi"("error in (no error)"=w750) -> ("error out"=w751:errorcluster)  [unwired: 5 in, 1 out]
        n635 = call <vilib>:"CloseHandle.vi"("client handle"=w745) -> ()  [unwired: 14 in, 1 out]
        n636 = call <vilib>:"Draw Flattened Pixmap.vi"("image data"=w740) -> ("new picture"=→"QQ登录二维码":picture)  [unwired: 8 in]
        n637 = call <vilib>:"General Error Handler.vi"("error in (no error)"=w751) -> ()  [unwired: 10 in, 5 out]
        n638 = UTF-8 to Text(11:w746) -> (3:w742:string)  [unwired: 2 in, 1 out]
        n639 = String Length(string=w742) -> (length=w743:i32)
        n640 = property on="webqq好友" class="Str"("Value"=w742) -> ()  [unwired: 2 in, 2 out]
        n641 = call <vilib>:"Clear Errors.vi"("error in (no error)"=w734) -> ("error out"=w735:errorcluster)  [unwired: 5 in, 1 out]
        n642 = Greater Than 0?(x=w743) -> (x > 0?=w741:bool)
        n643 = call <vilib>:"General Error Handler.vi"("error in (no error)"=w735) -> ()  [unwired: 10 in, 5 out]
        n644 = case shown="真" w741 {
          frame False {
          }
          frame True {
            w753 = T5."Enabled" ("禁用")
            w752 = FALSE ("获取好友标志")
            n645 = property on="接收者的QQ昵称或备注名" class="Str"("DisabledEnum"=w753) -> ()  [unwired: 2 in, 2 out]
            n646 = property on="搜索ID按钮" class="Bool"("DisabledEnum"=w753) -> ()  [unwired: 2 in, 2 out]
            n647 = property on="确认发送实时日志" class="Bool (严格)"("DisabledEnum"=w753) -> ()  [unwired: 2 in, 2 out]
            n648 = property on="退出QQ号按钮" class="Bool"("DisabledEnum"=w753) -> ()  [unwired: 2 in, 2 out]
            n649 = property on="正在加载标志" class="Bool (严格)"("Visible"=w752) -> ()  [unwired: 2 in, 2 out]
            "QQ状态" <- TRUE ("QQ状态")
            "正在加载标志" <- w752
          }
        }
      }
    }
  }
  n650 = while {
    stop <- FALSE stop-if-true
    # "选项卡切换"
    n651 = Current VI's Menubar() -> (w757:refnum<k9>)
    n652 = Get Menu Selection(0:w757) -> (6:w756:string)  [unwired: 3 in, 4 out]
    n653 = Wait (ms)(milliseconds to wait=u32 50 ("等待时间（毫秒）")) -> ()  [unwired: 1 out]
    n654 = case shown="\"关闭窗口\"" w756 {
      frame "假", Default {
      }
      frame "调试助手" {
        w759 = 1 ("禁用的索引 (列)")
        w782 = 0 ("禁用的索引 (列)")
        n655 = property on="清扫模式记录数组" class="Arr (严格)"() -> ("Value"=w774:dbl[][])  [unwired: 2 in, 2 out]
        n656 = Index Array(array=w774, index (row) #1=0 ("索引 (行)"), index (col) #1=w782, index (row) #2=1 ("索引 (行)"), index (col) #2=w782, index (row) #3=2 ("索引 (行)"), index (col) #3=w782, index (row) #4=3 ("索引 (行)"), index (col) #4=w782, index (row) #5=4 ("索引 (行)"), index (col) #5=w782, index (row) #6=5 ("索引 (行)"), index (col) #6=w782) -> (element #1=w775:dbl, element #2=w777:dbl, element #3=w783:dbl, element #4=w784:dbl, element #5=w785:dbl, element #6=w786:dbl)
        n657 = property on="晴类清扫周期：" class="Ring (严格)"("Value"=w775) -> ()  [unwired: 2 in, 2 out]
        n658 = property on="阴类清扫周期：" class="Ring (严格)"("Value"=w777) -> ()  [unwired: 2 in, 2 out]
        n659 = property on="雨类清扫周期：" class="Ring (严格)"("Value"=w783) -> ()  [unwired: 2 in, 2 out]
        n660 = property on="雪类清扫周期：" class="Ring (严格)"("Value"=w784) -> ()  [unwired: 2 in, 2 out]
        n661 = property on="沙尘类清扫周期：" class="Ring (严格)"("Value"=w785) -> ()  [unwired: 2 in, 2 out]
        n662 = property on="其他类清扫周期：" class="Ring (严格)"("Value"=w786) -> ()  [unwired: 2 in, 2 out]
        n663 = property on="清扫模式记录数组" class="Arr (严格)"() -> ("Value"=w765:dbl[][])  [unwired: 2 in, 2 out]
        n664 = property on="选项卡控件" class="TabCtl (严格)"("Value"=enum32{"主面板", "调试助手"}."调试助手" ("选项卡控件")) -> ()  [unwired: 2 in, 2 out]
        n665 = Index Array(array=w765, index (row) #1=0 ("索引 (行)"), index (col) #1=w759, index (row) #2=1 ("索引 (行)"), index (col) #2=w759, index (row) #3=2 ("索引 (行)"), index (col) #3=w759, index (row) #4=3 ("索引 (行)"), index (col) #4=w759, index (row) #5=4 ("索引 (行)"), index (col) #5=w759, index (row) #6=5 ("索引 (行)"), index (col) #6=w759) -> (element #1=w767:dbl, element #2=w768:dbl, element #3=w769:dbl, element #4=w770:dbl, element #5=w771:dbl, element #6=w772:dbl)
        n666 = property on="晴类清扫速度：" class="Slide (严格)"("Value"=w767) -> ()  [unwired: 2 in, 2 out]
        n667 = property on="阴类清扫速度：" class="Slide (严格)"("Value"=w768) -> ()  [unwired: 2 in, 2 out]
        n668 = property on="雨类清扫速度：" class="Slide (严格)"("Value"=w769) -> ()  [unwired: 2 in, 2 out]
        n669 = property on="雪类清扫速度：" class="Slide (严格)"("Value"=w770) -> ()  [unwired: 2 in, 2 out]
        n670 = property on="沙尘类清扫速度：" class="Slide (严格)"("Value"=w771) -> ()  [unwired: 2 in, 2 out]
        n671 = property on="其他类清扫速度：" class="Slide (严格)"("Value"=w772) -> ()  [unwired: 2 in, 2 out]
      }
      frame "保存配置" {
        n672 = flat-sequence {
          frame #0 {
            w788 = 1 ("禁用的索引 (列)")
            w811 = 0 ("禁用的索引 (列)")
            n673 = property on="清扫模式记录数组" class="Arr (严格)"() -> ("Value"=w803:dbl[][])  [unwired: 2 in, 2 out]
            n674 = property on="清扫模式记录数组" class="Arr (严格)"() -> ("Value"=w794:dbl[][])  [unwired: 2 in, 2 out]
            n675 = Index Array(array=w803, index (row) #1=0 ("索引 (行)"), index (col) #1=w811, index (row) #2=1 ("索引 (行)"), index (col) #2=w811, index (row) #3=2 ("索引 (行)"), index (col) #3=w811, index (row) #4=3 ("索引 (行)"), index (col) #4=w811, index (row) #5=4 ("索引 (行)"), index (col) #5=w811, index (row) #6=5 ("索引 (行)"), index (col) #6=w811) -> (element #1=w804:dbl, element #2=w806:dbl, element #3=w812:dbl, element #4=w813:dbl, element #5=w814:dbl, element #6=w815:dbl)
            n676 = Index Array(array=w794, index (row) #1=0 ("索引 (行)"), index (col) #1=w788, index (row) #2=1 ("索引 (行)"), index (col) #2=w788, index (row) #3=2 ("索引 (行)"), index (col) #3=w788, index (row) #4=3 ("索引 (行)"), index (col) #4=w788, index (row) #5=4 ("索引 (行)"), index (col) #5=w788, index (row) #6=5 ("索引 (行)"), index (col) #6=w788) -> (element #1=w796:dbl, element #2=w797:dbl, element #3=w798:dbl, element #4=w799:dbl, element #5=w800:dbl, element #6=w801:dbl)
            n677 = property on="晴类清扫周期：" class="Ring (严格)"("Value"=w804) -> ()  [unwired: 2 in, 2 out]
            n678 = property on="阴类清扫周期：" class="Ring (严格)"("Value"=w806) -> ()  [unwired: 2 in, 2 out]
            n679 = property on="雨类清扫周期：" class="Ring (严格)"("Value"=w812) -> ()  [unwired: 2 in, 2 out]
            n680 = property on="雪类清扫周期：" class="Ring (严格)"("Value"=w813) -> ()  [unwired: 2 in, 2 out]
            n681 = property on="沙尘类清扫周期：" class="Ring (严格)"("Value"=w814) -> ()  [unwired: 2 in, 2 out]
            n682 = property on="其他类清扫周期：" class="Ring (严格)"("Value"=w815) -> ()  [unwired: 2 in, 2 out]
            n683 = property on="晴类清扫速度：" class="Slide (严格)"("Value"=w796) -> ()  [unwired: 2 in, 2 out]
            n684 = property on="阴类清扫速度：" class="Slide (严格)"("Value"=w797) -> ()  [unwired: 2 in, 2 out]
            n685 = property on="雨类清扫速度：" class="Slide (严格)"("Value"=w798) -> ()  [unwired: 2 in, 2 out]
            n686 = property on="雪类清扫速度：" class="Slide (严格)"("Value"=w799) -> ()  [unwired: 2 in, 2 out]
            n687 = property on="沙尘类清扫速度：" class="Slide (严格)"("Value"=w800) -> ()  [unwired: 2 in, 2 out]
            n688 = property on="其他类清扫速度：" class="Slide (严格)"("Value"=w801) -> ()  [unwired: 2 in, 2 out]
          }
          frame #1 {
            n689 = property on="当前城市" class="Str"() -> ("Value"=w831:string)  [unwired: 2 in, 2 out]
            n690 = property on="雪类清扫速度：" class="Slide (严格)"() -> ("Value"=w821:i32)  [unwired: 2 in, 2 out]
            n691 = property on="沙尘类清扫速度：" class="Slide (严格)"() -> ("Value"=w822:i32)  [unwired: 2 in, 2 out]
            n692 = property on="其他类清扫速度：" class="Slide (严格)"() -> ("Value"=w823:i32)  [unwired: 2 in, 2 out]
            n693 = property on="阴类清扫速度：" class="Slide (严格)"() -> ("Value"=w824:i32)  [unwired: 2 in, 2 out]
            n694 = property on="其他类清扫周期：" class="Ring (严格)"() -> ("Value"=w825:dbl)  [unwired: 2 in, 2 out]
            n695 = property on="雪类清扫周期：" class="Ring (严格)"() -> ("Value"=w826:dbl)  [unwired: 2 in, 2 out]
            n696 = property on="阴类清扫周期：" class="Ring (严格)"() -> ("Value"=w827:dbl)  [unwired: 2 in, 2 out]
            n697 = property on="清扫模式选择开关" class="Bool (严格)"() -> ("Value"=w828:bool)  [unwired: 2 in, 2 out]
            n698 = property on="清扫速度：" class="Slide (严格)"() -> ("Value"=w829:i32)  [unwired: 2 in, 2 out]
            n699 = property on="清扫周期：" class="Ring (严格)"() -> ("Value"=w830:dbl)  [unwired: 2 in, 2 out]
            n700 = property on="晴类清扫周期：" class="Ring (严格)"() -> ("Value"=w816:dbl)  [unwired: 2 in, 2 out]
            n701 = property on="雨类清扫周期：" class="Ring (严格)"() -> ("Value"=w817:dbl)  [unwired: 2 in, 2 out]
            n702 = property on="沙尘类清扫周期：" class="Ring (严格)"() -> ("Value"=w818:dbl)  [unwired: 2 in, 2 out]
            n703 = property on="晴类清扫速度：" class="Slide (严格)"() -> ("Value"=w819:i32)  [unwired: 2 in, 2 out]
            n704 = property on="雨类清扫速度：" class="Slide (严格)"() -> ("Value"=w820:i32)  [unwired: 2 in, 2 out]
            n705 = property on="等待：" class="DigNum (严格)"() -> ("Value"=w832:i32)  [unwired: 2 in, 2 out]
            n706 = property on="端口号：" class="DigNum (严格)"() -> ("Value"=w833:i32)  [unwired: 2 in, 2 out]
            n707 = call "保存配置.vi"("端口号"=w833, "等待"=w832, "当前城市"=w831, "手动清扫周期"=w830, "手动清扫速度"=w829, "清扫模式选择开关"=w828, "晴类清扫周期"=w816, "阴类清扫周期"=w827, "雨类清扫周期"=w817, "雪类清扫周期"=w826, "沙尘类清扫周期"=w818, "其他类清扫周期"=w825, "晴类清扫速度"=w819, "阴类清扫速度"=w824, "雨类清扫速度"=w820, "雪类清扫速度"=w821, "沙尘类清扫速度"=w822, "其他类清扫速度"=w823) -> ()  [unwired: 2 in]
          }
        }
      }
      frame "读取配置" {
        n708 = flat-sequence {
          frame #0 {
            w834 = 1 ("禁用的索引 (列)")
            w857 = 0 ("禁用的索引 (列)")
            n709 = property on="清扫模式记录数组" class="Arr (严格)"() -> ("Value"=w840:dbl[][])  [unwired: 2 in, 2 out]
            n710 = property on="清扫模式记录数组" class="Arr (严格)"() -> ("Value"=w849:dbl[][])  [unwired: 2 in, 2 out]
            n711 = Index Array(array=w840, index (row) #1=0 ("索引 (行)"), index (col) #1=w834, index (row) #2=1 ("索引 (行)"), index (col) #2=w834, index (row) #3=2 ("索引 (行)"), index (col) #3=w834, index (row) #4=3 ("索引 (行)"), index (col) #4=w834, index (row) #5=4 ("索引 (行)"), index (col) #5=w834, index (row) #6=5 ("索引 (行)"), index (col) #6=w834) -> (element #1=w842:dbl, element #2=w843:dbl, element #3=w844:dbl, element #4=w845:dbl, element #5=w846:dbl, element #6=w847:dbl)
            n712 = Index Array(array=w849, index (row) #1=0 ("索引 (行)"), index (col) #1=w857, index (row) #2=1 ("索引 (行)"), index (col) #2=w857, index (row) #3=2 ("索引 (行)"), index (col) #3=w857, index (row) #4=3 ("索引 (行)"), index (col) #4=w857, index (row) #5=4 ("索引 (行)"), index (col) #5=w857, index (row) #6=5 ("索引 (行)"), index (col) #6=w857) -> (element #1=w850:dbl, element #2=w852:dbl, element #3=w858:dbl, element #4=w859:dbl, element #5=w860:dbl, element #6=w861:dbl)
            n713 = property on="晴类清扫速度：" class="Slide (严格)"("Value"=w842) -> ()  [unwired: 2 in, 2 out]
            n714 = property on="阴类清扫速度：" class="Slide (严格)"("Value"=w843) -> ()  [unwired: 2 in, 2 out]
            n715 = property on="雨类清扫速度：" class="Slide (严格)"("Value"=w844) -> ()  [unwired: 2 in, 2 out]
            n716 = property on="雪类清扫速度：" class="Slide (严格)"("Value"=w845) -> ()  [unwired: 2 in, 2 out]
            n717 = property on="沙尘类清扫速度：" class="Slide (严格)"("Value"=w846) -> ()  [unwired: 2 in, 2 out]
            n718 = property on="其他类清扫速度：" class="Slide (严格)"("Value"=w847) -> ()  [unwired: 2 in, 2 out]
            n719 = property on="晴类清扫周期：" class="Ring (严格)"("Value"=w850) -> ()  [unwired: 2 in, 2 out]
            n720 = property on="阴类清扫周期：" class="Ring (严格)"("Value"=w852) -> ()  [unwired: 2 in, 2 out]
            n721 = property on="雨类清扫周期：" class="Ring (严格)"("Value"=w858) -> ()  [unwired: 2 in, 2 out]
            n722 = property on="雪类清扫周期：" class="Ring (严格)"("Value"=w859) -> ()  [unwired: 2 in, 2 out]
            n723 = property on="沙尘类清扫周期：" class="Ring (严格)"("Value"=w860) -> ()  [unwired: 2 in, 2 out]
            n724 = property on="其他类清扫周期：" class="Ring (严格)"("Value"=w861) -> ()  [unwired: 2 in, 2 out]
          }
          frame #1 {
            n725 = call "读取配置.vi"() -> ("端口号"=w875:i32, "等待"=w874:i32, "当前城市"=w873:string, "手动清扫周期"=w872:dbl, "手动清扫速度"=w871:i32, "清扫模式选择开关"=w870:bool, "晴类清扫周期"=w876:dbl, "阴类清扫周期"=w869:dbl, "雨类清扫周期"=w877:dbl, "雪类清扫周期"=w868:dbl, "沙尘类清扫周期"=w878:dbl, "其他类清扫周期"=w867:dbl, "晴类清扫速度"=w879:i32, "阴类清扫速度"=w866:i32, "雨类清扫速度"=w862:i32, "雪类清扫速度"=w863:i32, "沙尘类清扫速度"=w864:i32, "其他类清扫速度"=w865:i32)  [unwired: 2 in]
            n726 = property on="当前城市" class="Str"("Value"=w873) -> ()  [unwired: 2 in, 2 out]
            n727 = property on="等待：" class="DigNum (严格)"("Value"=w874) -> ()  [unwired: 2 in, 2 out]
            n728 = property on="端口号：" class="DigNum (严格)"("Value"=w875) -> ()  [unwired: 2 in, 2 out]
            n729 = property on="雨类清扫速度：" class="Slide (严格)"("Value"=w862) -> ()  [unwired: 2 in, 2 out]
            n730 = property on="雪类清扫速度：" class="Slide (严格)"("Value"=w863) -> ()  [unwired: 2 in, 2 out]
            n731 = property on="沙尘类清扫速度：" class="Slide (严格)"("Value"=w864) -> ()  [unwired: 2 in, 2 out]
            n732 = property on="其他类清扫速度：" class="Slide (严格)"("Value"=w865) -> ()  [unwired: 2 in, 2 out]
            n733 = property on="阴类清扫速度：" class="Slide (严格)"("Value"=w866) -> ()  [unwired: 2 in, 2 out]
            n734 = property on="其他类清扫周期：" class="Ring (严格)"("Value"=w867) -> ()  [unwired: 2 in, 2 out]
            n735 = property on="雪类清扫周期：" class="Ring (严格)"("Value"=w868) -> ()  [unwired: 2 in, 2 out]
            n736 = property on="阴类清扫周期：" class="Ring (严格)"("Value"=w869) -> ()  [unwired: 2 in, 2 out]
            n737 = property on="清扫模式选择开关" class="Bool (严格)"("Value"=w870) -> ()  [unwired: 2 in, 2 out]
            n738 = property on="清扫速度：" class="Slide (严格)"("Value"=w871) -> ()  [unwired: 2 in, 2 out]
            n739 = property on="清扫周期：" class="Ring (严格)"("Value"=w872) -> ()  [unwired: 2 in, 2 out]
            n740 = property on="晴类清扫周期：" class="Ring (严格)"("Value"=w876) -> ()  [unwired: 2 in, 2 out]
            n741 = property on="雨类清扫周期：" class="Ring (严格)"("Value"=w877) -> ()  [unwired: 2 in, 2 out]
            n742 = property on="沙尘类清扫周期：" class="Ring (严格)"("Value"=w878) -> ()  [unwired: 2 in, 2 out]
            n743 = property on="晴类清扫速度：" class="Slide (严格)"("Value"=w879) -> ()  [unwired: 2 in, 2 out]
          }
        }
      }
      frame "主面板" {
        n744 = flat-sequence {
          frame #0 {
            n745 = disable-structure shown="禁用" {
              frame Disabled {
                n746 = property on="天气：" class="Str"() -> ("Value"=w888:string)  [unwired: 2 in, 2 out]
                n747 = Concatenate Strings("和风天气图标\\" ("字符串"), w888, ".png" ("字符串")) -> (w885:string)
                n748 = call <vilib>:"Application Directory.vi"() -> ("Application Directory"=w886:path)
                n749 = Build Path(base path=w886, name or relative path=w885) -> (appended path=w887:path)
                n750 = call "显示图片.vi"("路径"=w887, "缩放因子"=1.1) -> ("二维图片"=w881:T2)  [unwired: 8 in]
                n751 = property on="天气图标" class="Pict (严格)"("Value"=w881) -> ()  [unwired: 2 in, 2 out]
              }
              frame Enabled {
              }
            }
          }
          frame #1 {
            w898 = 0 ("禁用的索引 (列)")
            w916 = 1 ("禁用的索引 (列)")
            n752 = property on="清扫模式记录数组" class="Arr (严格)"() -> ("Value"=w890:dbl[][])  [unwired: 2 in, 2 out]
            n753 = property on="清扫模式记录数组" class="Arr (严格)"() -> ("Value"=w910:dbl[][])  [unwired: 2 in, 2 out]
            n754 = Index Array(array=w890, index (row) #1=0 ("索引 (行)"), index (col) #1=w898, index (row) #2=1 ("索引 (行)"), index (col) #2=w898, index (row) #3=2 ("索引 (行)"), index (col) #3=w898, index (row) #4=3 ("索引 (行)"), index (col) #4=w898, index (row) #5=4 ("索引 (行)"), index (col) #5=w898, index (row) #6=5 ("索引 (行)"), index (col) #6=w898) -> (element #1=w891:dbl, element #2=w893:dbl, element #3=w899:dbl, element #4=w900:dbl, element #5=w901:dbl, element #6=w902:dbl)
            n755 = Index Array(array=w910, index (row) #1=0 ("索引 (行)"), index (col) #1=w916, index (row) #2=1 ("索引 (行)"), index (col) #2=w916, index (row) #3=2 ("索引 (行)"), index (col) #3=w916, index (row) #4=3 ("索引 (行)"), index (col) #4=w916, index (row) #5=4 ("索引 (行)"), index (col) #5=w916, index (row) #6=5 ("索引 (行)"), index (col) #6=w916) -> (element #1=w908:dbl, element #2=w907:dbl, element #3=w906:dbl, element #4=w905:dbl, element #5=w904:dbl, element #6=w903:dbl)
            n756 = property on="晴类清扫周期：" class="Ring (严格)"("Value"=w891) -> ()  [unwired: 2 in, 2 out]
            n757 = property on="阴类清扫周期：" class="Ring (严格)"("Value"=w893) -> ()  [unwired: 2 in, 2 out]
            n758 = property on="雨类清扫周期：" class="Ring (严格)"("Value"=w899) -> ()  [unwired: 2 in, 2 out]
            n759 = property on="雪类清扫周期：" class="Ring (严格)"("Value"=w900) -> ()  [unwired: 2 in, 2 out]
            n760 = property on="沙尘类清扫周期：" class="Ring (严格)"("Value"=w901) -> ()  [unwired: 2 in, 2 out]
            n761 = property on="其他类清扫周期：" class="Ring (严格)"("Value"=w902) -> ()  [unwired: 2 in, 2 out]
            n762 = property on="晴类清扫速度：" class="Slide (严格)"("Value"=w908) -> ()  [unwired: 2 in, 2 out]
            n763 = property on="阴类清扫速度：" class="Slide (严格)"("Value"=w907) -> ()  [unwired: 2 in, 2 out]
            n764 = property on="雨类清扫速度：" class="Slide (严格)"("Value"=w906) -> ()  [unwired: 2 in, 2 out]
            n765 = property on="雪类清扫速度：" class="Slide (严格)"("Value"=w905) -> ()  [unwired: 2 in, 2 out]
            n766 = property on="沙尘类清扫速度：" class="Slide (严格)"("Value"=w904) -> ()  [unwired: 2 in, 2 out]
            n767 = property on="其他类清扫速度：" class="Slide (严格)"("Value"=w903) -> ()  [unwired: 2 in, 2 out]
          }
        }
        n768 = property on="选项卡控件" class="TabCtl (严格)"("Value"=enum32{"主面板", "调试助手"}."主面板" ("选项卡控件")) -> ()  [unwired: 2 in, 2 out]
      }
      frame "清扫模式设置" {
        w917 = 1 ("禁用的索引 (列)")
        w940 = 0 ("禁用的索引 (列)")
        n769 = property on="清扫模式记录数组" class="Arr (严格)"() -> ("Value"=w932:dbl[][])  [unwired: 2 in, 2 out]
        n770 = Index Array(array=w932, index (row) #1=0 ("索引 (行)"), index (col) #1=w940, index (row) #2=1 ("索引 (行)"), index (col) #2=w940, index (row) #3=2 ("索引 (行)"), index (col) #3=w940, index (row) #4=3 ("索引 (行)"), index (col) #4=w940, index (row) #5=4 ("索引 (行)"), index (col) #5=w940, index (row) #6=5 ("索引 (行)"), index (col) #6=w940) -> (element #1=w933:dbl, element #2=w935:dbl, element #3=w941:dbl, element #4=w942:dbl, element #5=w943:dbl, element #6=w944:dbl)
        n771 = property on="晴类清扫周期：" class="Ring (严格)"("Value"=w933) -> ()  [unwired: 2 in, 2 out]
        n772 = property on="阴类清扫周期：" class="Ring (严格)"("Value"=w935) -> ()  [unwired: 2 in, 2 out]
        n773 = property on="雨类清扫周期：" class="Ring (严格)"("Value"=w941) -> ()  [unwired: 2 in, 2 out]
        n774 = property on="雪类清扫周期：" class="Ring (严格)"("Value"=w942) -> ()  [unwired: 2 in, 2 out]
        n775 = property on="沙尘类清扫周期：" class="Ring (严格)"("Value"=w943) -> ()  [unwired: 2 in, 2 out]
        n776 = property on="其他类清扫周期：" class="Ring (严格)"("Value"=w944) -> ()  [unwired: 2 in, 2 out]
        n777 = property on="选项卡控件" class="TabCtl (严格)"("Value"=enum32{"主面板", "调试助手", "清扫模式设置"}."清扫模式设置" ("选项卡控件")) -> ()  [unwired: 2 in, 2 out]
        n778 = property on="清扫模式记录数组" class="Arr (严格)"() -> ("Value"=w923:dbl[][])  [unwired: 2 in, 2 out]
        n779 = Index Array(array=w923, index (row) #1=0 ("索引 (行)"), index (col) #1=w917, index (row) #2=1 ("索引 (行)"), index (col) #2=w917, index (row) #3=2 ("索引 (行)"), index (col) #3=w917, index (row) #4=3 ("索引 (行)"), index (col) #4=w917, index (row) #5=4 ("索引 (行)"), index (col) #5=w917, index (row) #6=5 ("索引 (行)"), index (col) #6=w917) -> (element #1=w925:dbl, element #2=w926:dbl, element #3=w927:dbl, element #4=w928:dbl, element #5=w929:dbl, element #6=w930:dbl)
        n780 = property on="晴类清扫速度：" class="Slide (严格)"("Value"=w925) -> ()  [unwired: 2 in, 2 out]
        n781 = property on="阴类清扫速度：" class="Slide (严格)"("Value"=w926) -> ()  [unwired: 2 in, 2 out]
        n782 = property on="雨类清扫速度：" class="Slide (严格)"("Value"=w927) -> ()  [unwired: 2 in, 2 out]
        n783 = property on="雪类清扫速度：" class="Slide (严格)"("Value"=w928) -> ()  [unwired: 2 in, 2 out]
        n784 = property on="沙尘类清扫速度：" class="Slide (严格)"("Value"=w929) -> ()  [unwired: 2 in, 2 out]
        n785 = property on="其他类清扫速度：" class="Slide (严格)"("Value"=w930) -> ()  [unwired: 2 in, 2 out]
      }
      frame "使用说明" {
        n786 = property on="选项卡控件" class="TabCtl (严格)"("Value"=enum32{"主面板", "调试助手", "清扫模式设置", "使用说明", "关于软件"}."使用说明" ("选项卡控件")) -> ()  [unwired: 2 in, 2 out]
        n787 = invoke on="调用节点" class="IWebBrowser2" method="Navigate2"(reference="WebBrowser", "URL"="https://skkkyoyo.github.io/Controller-of-solar-roof-cleaning-robot/") -> ()  [unwired: 6 in, 8 out]
      }
      frame "关闭窗口" {
        n788 = stacked-sequence {
          frame #0 {
            n789 = property on="正在加载标志" class="Bool (严格)"("Value"=FALSE ("获取好友标志")) -> ()  [unwired: 2 in, 2 out]
            n790 = property on="QQ状态" class="Bool (严格)"("Value"=FALSE ("QQ状态")) -> ()  [unwired: 2 in, 2 out]
            n791 = property on="webqq好友" class="Str"() -> ("Value"=w960:string)  [unwired: 2 in, 2 out]
            n792 = Match Pattern(string=w960, regular expression="\"id\":" ("正则表达式")) -> (after substring=w968:string)  [unwired: 1 in, 3 out]
            n793 = call <vilib>:"Application Directory.vi"() -> ("Application Directory"=w950:path)
            n794 = call <vilib>:"Application Directory.vi"() -> ("Application Directory"=w957:path)
            n795 = Match Pattern(string=w968, regular expression="," ("正则表达式")) -> (before substring=w970:string)  [unwired: 1 in, 3 out]
            n796 = Build Path(base path=w950, name or relative path="Mojo-StrawberryPerl\\tmp\\mojo_webqq_cookie_default.dat" ("名称或相对路径")) -> (appended path=w952:path)
            n797 = Build Path(base path=w957, name or relative path="Mojo-StrawberryPerl\\tmp\\mojo_webqq_state_default.json" ("名称或相对路径")) -> (appended path=w955:path)
            n798 = call <vilib>:"Check if File or Folder Exists.vi"("path"=w952) -> ("file or folder exists?"=w953:bool, "dup path"=w954:path)  [unwired: 8 in, 1 out]
            n799 = call <vilib>:"Check if File or Folder Exists.vi"("path"=w955) -> ("file or folder exists?"=w958:bool, "dup path"=w959:path)  [unwired: 8 in, 1 out]
            n800 = Concatenate Strings("http://127.0.0.1:5000/openqq/send_friend_message?id=" ("字符串"), w970, "&content=!stop!" ("字符串")) -> (w966:string)
            n801 = case shown="真" w958 {
              tunnel: w959 -> [_ w974]
              frame False {
              }
              frame True {
                n802 = Delete(path (use dialog)=w974) -> ()  [unwired: 4 in, 3 out]
              }
            }
            n803 = case shown="真" w953 {
              tunnel: w954 -> [_ w975]
              frame False {
              }
              frame True {
                n804 = Delete(path (use dialog)=w975) -> ()  [unwired: 4 in, 3 out]
              }
            }
            n805 = call <vilib>:"OpenHandle.vi"() -> ("client handle out"=w962:T7)  [unwired: 14 in, 1 out]
            n806 = Text to UTF-8(11:w966) -> (3:w963:string)  [unwired: 2 in, 1 out]
            n807 = call <vilib>:"GET.vi"("client handle"=w962, "url"=w963) -> ("client handle out"=w961:T7, "error out"=w964:errorcluster)  [unwired: 10 in, 2 out]
            n808 = call <vilib>:"CloseHandle.vi"("client handle"=w961) -> ()  [unwired: 14 in, 1 out]
            n809 = call <vilib>:"Clear Errors.vi"("error in (no error)"=w964) -> ()  [unwired: 5 in, 2 out]
            n810 = call <vilib>:"General Error Handler.vi"() -> ()  [unwired: 11 in, 5 out]
            n811 = Wait (ms)(milliseconds to wait=u32 1000 ("等待时间（毫秒）")) -> ()  [unwired: 1 out]
          }
          frame #1 {
            n812 = Stop(stop? (T)=TRUE ("停止？(T)")) -> ()
          }
        }
      }
      frame "检查更新" {
        n813 = call <vilib>:"System Exec.vi"("run minimized? (F)"=TRUE, "command line"="CMD /C start https://skkkyoyo.github.io/Controller-of-solar-roof-cleaning-robot/") -> ()  [unwired: 6 in, 4 out]
      }
      frame "实时日志发送" {
        n814 = property on="选项卡控件" class="TabCtl (严格)"("Value"=T1."实时日志发送" ("选项卡控件")) -> ()  [unwired: 2 in, 2 out]
      }
      frame "关于软件" {
        n815 = property on="选项卡控件" class="TabCtl (严格)"("Value"=enum32{"主面板", "调试助手", "清扫模式设置", "使用说明", "关于软件"}."关于软件" ("选项卡控件")) -> ()  [unwired: 2 in, 2 out]
      }
    }
  }
  n816 = while {
    i -> [w983]
    stop <- FALSE stop-if-true
    n817 = Quotient & Remainder(x=w983, y=200) -> (x-y*floor(x/y)=w982:i32)  [unwired: 1 out]
    n818 = Greater?(x=w982, y=99) -> (0:w981:bool)
    n819 = Wait (ms)(milliseconds to wait=u32 20 ("等待时间（毫秒）")) -> ()  [unwired: 1 out]
    n820 = case shown="真" w981 {
      tunnel: w982 -> [w988 w989]
      frame False {
        "滑动杆" <- w988
      }
      frame True {
        n821 = Subtract(x=u32 200 ("等待时间（毫秒）"), y=w989) -> (x-y=w990:u32)
        n822 = property on="滑动杆" class="Slide (严格)"("Value"=w990) -> ()  [unwired: 2 in, 2 out]
      }
    }
  }
  n823 = TCP Close Connection(connection ID=w1) -> ()  [unwired: 2 in, 2 out]
  n824 = while {
    stop <- FALSE stop-if-true
    n825 = call "获取时间.vi"() -> ("当前小时数"=w992:string)  [unwired: 8 in, 3 out]
    n826 = property on="测试布尔" class="Bool (严格)"() -> ("Value"=w1003:bool)  [unwired: 2 in, 2 out]
    n827 = property on="起始小时" class="Str"() -> ("Value"=w997:string)  [unwired: 2 in, 2 out]
    n828 = Not(x=w1003) -> (.not. x?=→"测试布尔":bool)
    n829 = Decimal String To Number(string=w992) -> (number=w996:i32)  [unwired: 2 in, 1 out]
    n830 = Decimal String To Number(string=w997) -> (number=w998:i32)  [unwired: 2 in, 1 out]
    n831 = Subtract(x=w996, y=w998) -> (x-y=w999:i32)
    n832 = Wait (ms)(milliseconds to wait=u32 50 ("等待时间（毫秒）")) -> ()  [unwired: 1 out]
    n833 = Absolute Value(x=w999) -> (abs(x)=w1000:i32)
    n834 = Quotient & Remainder(x=w1000, y=24) -> (x-y*floor(x/y)=w995:i32)  [unwired: 1 out]
    n835 = Equal?(x=w995, y=4) -> (x = y?=w993:bool)
    n836 = case shown="真" w993 {
      frame False {
      }
      frame True {
        n837 = property on="清扫模式选择开关" class="Bool (严格)"() -> ("Value"=w1007:bool)  [unwired: 2 in, 2 out]
        n838 = property on="连接状态" class="Bool (严格)"() -> ("Value"=w1008:bool)  [unwired: 2 in, 2 out]
        n839 = And(x=w1008, y=w1007) -> (x .and. y?=w1006:bool)
        n840 = flat-sequence {
          frame #0 {
            n841 = property on="当前城市" class="Str"() -> ("Value"=w1010:string)  [unwired: 2 in, 2 out]
            n842 = call "抓取天气查询.vi"("城市（市，县）"=w1010) -> ("当前天气"=w1009:string)
            n843 = property on="天气：" class="Str"("Value"=w1009) -> ()  [unwired: 2 in, 2 out]
            n844 = Wait (ms)(milliseconds to wait=u32 500 ("等待时间（毫秒）")) -> ()  [unwired: 1 out]
          }
          frame #1 {
            n845 = property on="天气：" class="Str"() -> ("Value"=w1012:string)  [unwired: 2 in, 2 out]
            n846 = Concatenate Strings("和风天气图标\\" ("字符串"), w1012, ".png" ("字符串")) -> (w1016:string)
            n847 = call <vilib>:"Application Directory.vi"() -> ("Application Directory"=w1015:path)
            n848 = Build Path(base path=w1015, name or relative path=w1016) -> (appended path=w1014:path)
            n849 = call "显示图片.vi"("路径"=w1014, "缩放因子"=1.1) -> ("二维图片"=w1013:T2)  [unwired: 8 in]
            n850 = property on="天气图标" class="Pict (严格)"("Value"=w1013) -> ()  [unwired: 2 in, 2 out]
          }
        }
        n851 = case shown="真" w1006 {
          frame False {
            # "如果为手动则不需要更改清理周期及速度"
            # "手动清扫模式"
          }
          frame True {
            # "智能清扫模式"
            n852 = flat-sequence {
              frame #0 {
                # "处理清扫周期"
                n853 = property on="天气：" class="Str"() -> ("Value"=w1037:string)  [unwired: 2 in, 2 out]
                n854 = case shown="\"薄雾\", \"多云\", \"少云\", \"雾\", \"阴\", \"霾\"" w1037 {
                  frame "假", Default {
                    n855 = property on="清扫模式记录数组" class="Arr (严格)"() -> ("Value"=w1041:dbl[][])  [unwired: 2 in, 2 out]
                    n856 = Index Array(array=w1041, index (row)=5 ("索引 (行)"), index (col)=0 ("禁用的索引 (列)")) -> (element=w1038:dbl)
                    n857 = property on="定时数" class="DigNum (严格)"("Value"=w1038) -> ()  [unwired: 2 in, 2 out]
                  }
                  frame "晴", "晴间多云" {
                    # "晴类"
                    n858 = property on="清扫模式记录数组" class="Arr (严格)"() -> ("Value"=w1045:dbl[][])  [unwired: 2 in, 2 out]
                    n859 = Index Array(array=w1045, index (row)=0 ("索引 (行)"), index (col)=0 ("禁用的索引 (列)")) -> (element=w1042:dbl)
                    n860 = property on="定时数" class="DigNum (严格)"("Value"=w1042) -> ()  [unwired: 2 in, 2 out]
                  }
                  frame "薄雾", "多云", "少云", "雾", "阴", "霾" {
                    # "阴类"
                    n861 = property on="清扫模式记录数组" class="Arr (严格)"() -> ("Value"=w1049:dbl[][])  [unwired: 2 in, 2 out]
                    n862 = Index Array(array=w1049, index (row)=1 ("索引 (行)"), index (col)=0 ("禁用的索引 (列)")) -> (element=w1046:dbl)
                    n863 = property on="定时数" class="DigNum (严格)"("Value"=w1046) -> ()  [unwired: 2 in, 2 out]
                  }
                  frame "暴雨", "大暴雨", "大雨", "极端降雨", "雷阵雨", "毛毛雨", "强雷阵雨", "强阵雨", "特大暴雨", "细雨", "小雨", "阵雨", "中雨" {
                    # "雨类"
                    n864 = property on="清扫模式记录数组" class="Arr (严格)"() -> ("Value"=w1053:dbl[][])  [unwired: 2 in, 2 out]
                    n865 = Index Array(array=w1053, index (row)=2 ("索引 (行)"), index (col)=0 ("禁用的索引 (列)")) -> (element=w1050:dbl)
                    n866 = property on="定时数" class="DigNum (严格)"("Value"=w1050) -> ()  [unwired: 2 in, 2 out]
                  }
                  frame "暴雪", "大雪", "冻雨", "雷阵雨伴有冰雹", "小雪", "雨夹雪", "雨雪天气", "阵雪", "阵雨夹雪", "中雪" {
                    # "雪类"
                    n867 = property on="清扫模式记录数组" class="Arr (严格)"() -> ("Value"=w1054:dbl[][])  [unwired: 2 in, 2 out]
                    n868 = Index Array(array=w1054, index (row)=3 ("索引 (行)"), index (col)=0 ("禁用的索引 (列)")) -> (element=w1055:dbl)
                    n869 = property on="定时数" class="DigNum (严格)"("Value"=w1055) -> ()  [unwired: 2 in, 2 out]
                  }
                  frame "浮尘", "龙卷风", "强沙尘暴", "沙尘暴", "扬沙" {
                    # "沙尘类"
                    n870 = property on="清扫模式记录数组" class="Arr (严格)"() -> ("Value"=w1061:dbl[][])  [unwired: 2 in, 2 out]
                    n871 = Index Array(array=w1061, index (row)=4 ("索引 (行)"), index (col)=0 ("禁用的索引 (列)")) -> (element=w1058:dbl)
                    n872 = property on="定时数" class="DigNum (严格)"("Value"=w1058) -> ()  [unwired: 2 in, 2 out]
                  }
                }
              }
              frame #1 {
                n873 = property on="定时数" class="DigNum (严格)"() -> ("Value"=w1066:dbl)  [unwired: 2 in, 2 out]
                n874 = Number To Fractional String(number=w1066, precision (6)=i16 1 ("精度(6)")) -> (F-format string=w1064:string)  [unwired: 2 in]
                n875 = Concatenate Strings(w1064, "小时" ("字符串")) -> (w1063:string)
                n876 = property on="清扫周期：" class="Str"("Value"=w1063) -> ()  [unwired: 2 in, 2 out]
              }
            }
            n877 = property on="刷新标志" class="Bool (严格)"("Value"=TRUE ("刷新标志")) -> ()  [unwired: 2 in, 2 out]
            n878 = disable-structure shown="禁用" {
              frame Disabled {
                n879 = property on="天气：" class="Str"() -> ("Value"=w1026:string)  [unwired: 2 in, 2 out]
                n880 = case shown="\"浮尘\", \"龙卷风\", \"强沙尘暴\", \"沙尘暴\", \"扬沙\"" w1026 {
                  tunnel: [w1031 w1032 w1033 w1034 w1035 w1036] -> w1030
                  frame "假", Default {
                    # "其他"
                    n881 = property on="其他类清扫速度：" class="Slide (严格)"() -> ("Value"=w1031:i32)  [unwired: 2 in, 2 out]
                  }
                  frame "晴", "晴间多云" {
                    # "晴类"
                    n882 = property on="晴类清扫速度：" class="Slide (严格)"() -> ("Value"=w1032:i32)  [unwired: 2 in, 2 out]
                  }
                  frame "薄雾", "多云", "少云", "雾", "阴", "霾" {
                    # "阴类"
                    n883 = property on="阴类清扫速度：" class="Slide (严格)"() -> ("Value"=w1033:i32)  [unwired: 2 in, 2 out]
                  }
                  frame "暴雨", "大暴雨", "大雨", "极端降雨", "雷阵雨", "毛毛雨", "强雷阵雨", "强阵雨", "特大暴雨", "细雨", "小雨", "阵雨", "中雨" {
                    # "雨类"
                    n884 = property on="雨类清扫速度：" class="Slide (严格)"() -> ("Value"=w1034:i32)  [unwired: 2 in, 2 out]
                  }
                  frame "暴雪", "大雪", "冻雨", "雷阵雨伴有冰雹", "小雪", "雨夹雪", "雨雪天气", "阵雪", "阵雨夹雪", "中雪" {
                    # "雪类"
                    n885 = property on="雪类清扫速度：" class="Slide (严格)"() -> ("Value"=w1035:i32)  [unwired: 2 in, 2 out]
                  }
                  frame "浮尘", "龙卷风", "强沙尘暴", "沙尘暴", "扬沙" {
                    # "沙尘类"
                    n886 = property on="沙尘类清扫速度：" class="Slide (严格)"() -> ("Value"=w1036:i32)  [unwired: 2 in, 2 out]
                  }
                }
                n887 = formula code="Y=X*15+105;"("X"=w1030) -> ("Y"=w1027:dbl)
                n888 = Number To Decimal String(number=w1027) -> (decimal integer string=w1029:string)  [unwired: 1 in]
                n889 = Concatenate Strings("pwm" ("字符串"), w1029) -> (w1024:string)
                n890 = property on="清扫速度：" class="Str"("Value"=w1024) -> ()  [unwired: 2 in, 2 out]
                n891 = TCP Write(data in=w1024) -> (connection ID out=w1023:refnum<k5>, error out=w1022:errorcluster)  [unwired: 3 in, 1 out]
                n892 = TCP Close Connection(connection ID=w1023, error in (no error)=w1022) -> (error out=w1021:errorcluster)  [unwired: 1 in, 1 out]
                n893 = call <vilib>:"Clear Errors.vi"("error in (no error)"=w1021) -> ("error out"=w1025:errorcluster)  [unwired: 5 in, 1 out]
                n894 = call <vilib>:"Simple Error Handler.vi"("error in (no error)"=w1025) -> ()  [unwired: 4 in, 5 out]
              }
              frame Enabled {
              }
            }
          }
        }
      }
    }
  }
  n895 = while {
    stop <- FALSE stop-if-true
    # "获取天气"
    n896 = property on="天气：" class="Str"() -> ("Value"=w1074:string)  [unwired: 2 in, 2 out]
    n897 = property on="当前城市" class="Str"() -> ("Value"=w1070:string)  [unwired: 2 in, 2 out]
    n898 = Equal?(x=w1074, y="") -> (x = y?=w1071:bool)
    n899 = Wait (ms)(milliseconds to wait=u32 20 ("等待时间（毫秒）")) -> ()  [unwired: 1 out]
    n900 = Not Equal?(x=w1070, y="") -> (x != y?=w1068:bool)
    n901 = And(x=w1071, y=w1068) -> (x .and. y?=w1067:bool)
    n902 = Or(x="确定当前城市", y=w1067) -> (x .or. y?=w1072:bool)
    n903 = case shown="真" w1072 {
      frame False {
      }
      frame True {
        n904 = flat-sequence {
          frame #0 {
            n905 = call "抓取天气查询.vi"("城市（市，县）"="当前城市") -> ("当前天气"=→"天气：":string)
            n906 = Wait (ms)(milliseconds to wait=u32 20 ("等待时间（毫秒）")) -> ()  [unwired: 1 out]
          }
          frame #1 {
            n907 = property on="天气：" class="Str"() -> ("Value"=w1083:string)  [unwired: 2 in, 2 out]
            n908 = property on="清扫模式选择开关" class="Bool (严格)"() -> ("Value"=w1081:bool)  [unwired: 2 in, 2 out]
            n909 = case shown="真" w1081 {
              frame False {
              }
              frame True {
                n910 = property on="清扫模式选择开关" class="Bool (严格)"("Val(Sgnl)"=TRUE ("值(信号)")) -> ()  [unwired: 2 in, 2 out]
              }
            }
            n911 = case shown="\"\"" w1083 {
              tunnel: [w1092 "未知" ("字符串")] -> w1082
              frame "假", Default {
                n912 = property on="天气：" class="Str"() -> ("Value"=w1092:string)  [unwired: 2 in, 2 out]
              }
              frame "" {
              }
            }
            n913 = Concatenate Strings("和风天气图标\\" ("字符串"), w1082, ".png" ("字符串")) -> (w1086:string)
            n914 = call <vilib>:"Application Directory.vi"() -> ("Application Directory"=w1085:path)
            n915 = Build Path(base path=w1085, name or relative path=w1086) -> (appended path=w1084:path)
            "图片路径" <- w1084
            n916 = call "显示图片.vi"("路径"=w1084, "缩放因子"=1.1) -> ("二维图片"=→"天气图标":T2)  [unwired: 8 in]
          }
        }
      }
    }
  }
  n917 = while {
    stop <- FALSE stop-if-true
    # "一分钟定时"
    n918 = property on="控制器IP：" class="Str"() -> ("Value"=w1096:string)  [unwired: 2 in, 2 out]
    n919 = String Length(string=w1096) -> (length=w1095:i32)
    n920 = Greater Than 0?(x=w1095) -> (x > 0?=w1094:bool)
    n921 = case shown="真" w1094 {
      frame False {
      }
      frame True {
        n922 = flat-sequence {
          frame #0 {
            n923 = Multiply(x="定时数", y=10.0) -> (x*y=w1098:dbl)
            n924 = for {
              N: w1098 -> [w1105]
              stop <- w1104 continue-if-true
              n925 = property on="定时数" class="DigNum (严格)"() -> ("Value"=w1103:dbl)  [unwired: 2 in, 2 out]
              n926 = Wait Until Next ms Multiple(millisecond multiple=u32 1000 ("毫秒倍数")) -> ()  [unwired: 1 out]
              n927 = Multiply(x=w1103, y=10.0) -> (x*y=w1101:dbl)
              n928 = Equal?(x=w1105, y=w1101) -> (x = y?=w1104:bool)
              "修改定时数标志" <- w1104
            }
          }
          frame #1 {
            n929 = property on="修改定时数标志" class="Bool (严格)"() -> ("Value"=w1107:bool)  [unwired: 2 in, 2 out]
            n930 = case shown="假" w1107 {
              frame False {
                n931 = property on="定时数" class="DigNum (严格)"() -> ("Value"=w1112:dbl)  [unwired: 2 in, 2 out]
                n932 = Number To Fractional String(use system decimal point (T)=TRUE ("使用系统小数点(T)"), number=w1112, precision (6)=i16 1 ("精度(6)")) -> (F-format string=w1108:string)  [unwired: 1 in]
                n933 = Concatenate Strings(w1108, "小时" ("字符串")) -> (w1113:string)
                n934 = property on="清扫周期：" class="Str"("Value"=w1113) -> ()  [unwired: 2 in, 2 out]
              }
              frame True {
                "清扫命令发出标志" <- TRUE ("清扫命令发出")
              }
            }
          }
        }
      }
    }
  }
